vi "Striptest.vi"(1 "Simulation?":bool) -> ()   [LabVIEW 2013]
uses:
  InstrControl/SupplyControl/SupplyControl.lvclass
  InstrControl/Switching/Switching.lvclass
  InstrControl/ProbeStationControl/ProbeStationControl.lvclass
  InstrControl/LCRControl/LCRControl.lvclass
  general_VIs/globals/QC_MeasurementSetup.vi
  striptest/ProbePlan/ProbePlanParams.vi
  general_VIs/globals/QC_RunInformation.vi
  InstrControl/InstrumentSetup.vi
  <vilib>/regexp/Match Regular Expression.xnode
  InstrControl/InstrControl.lvclass
  InstrControl/ArduinoControl/ArduinoControl.lvclass
  <vilib>/Analysis/NI_AALBase.lvlib
panel:
  out "Tab Control":enum32{"Striptest Setup", "Striptest"}(tab)
  in  "Bias Voltage [V]":dbl=-150.0 format="%.1f"
  in  "Frequency [Hz] Setup":i32=1000 caption="Frequency [Hz]" format="%#.3p"
  in  "Minimum fraction\nof good strips":dbl=98.0 format="%.1g"
  in  "Quit":bool
  in  "Continue":bool
  in  "Measurement Configurations":bool
  in  "Pinholes Y/N":bool=TRUE
  in  "Capacitance Y/N":bool=TRUE
  in  "Resistance Y/N":bool=TRUE
  in  "Striptest SMU":string(combo)="Keithley 2410"
  in  "LCR Meter":string(combo)="WayneKerr 6440B"
  in  "Temperature":enum16{"Read Arduino", "Enter manually"}(ring)
  in  "Bias Supply":string(combo)="Keithley 2410"
  in  "Hardware Configurations":bool
  in  "DB Serial No. IN:":string caption="DB Serial No.:"
  in  "User:":string(combo)="Christoph"
  in  "Batch No. IN:":string caption="Batch No.:"
  in  "Device Category IN:":string(combo)="Short Strip" caption="Device Category:"
  in  "Sensor Serial No. IN:":string caption="Sensor Serial No.:"
  in  "From4":u16(ring)
  in  "From3":u16(ring)
  in  "From2":u16(ring)
  in  "From 1":u16(ring) caption="From"
  in  "To4":u16(ring)
  in  "To3":u16(ring)
  in  "To2":u16(ring)
  in  "To 1":u16(ring) caption="To"
  out "Region 1":string caption="Region"
  out "Region2":string
  out "Region3":string
  out "Region4":string
  in  "Enable1":bool
  in  "Enable4":bool
  in  "Enable2":bool
  in  "Enable3":bool
  in  "Pinhole Parameters IN":T1={"Base Voltage"=10.0, "Base Ramp [V/step]"=10.0, "Base Step [ms]"=1000, "High Voltage"=100.0, "High Ramp [V/step]"=100.0, "High Step [ms]"=1000} caption="Pinhole Measurement Parameters"
  in  "Manufacturer:":string(combo)="Hamamatsu"
  in  "Auto ReCheck":bool
  in  "Thresholds:":T2={"Current [nA]"=200.0, "Ccoupl Lo [pF/cm]"=20.0, "Ccoupl Hi [pF/cm]"=33.0, "Rbias Lo [MW]"=1.0, "Rbias Hi [MW]"=2.0}
  in  "Rolling\nCurrent Readout":bool=TRUE
  in  "settling\ndelay [ms]":i32=50
  in  "Pinhole Parameters":T1={"Base Voltage"=10.0, "Base Ramp [V/step]"=10.0, "Base Step [ms]"=1000, "High Voltage"=100.0, "High Ramp [V/step]"=100.0, "High Step [ms]"=1000}
  out "Bias On/Off:":bool
  in  "Auto quit &\nswitch off bias":bool
  out "Sensor No.:":string
  out "Device Category:":string
  out "DB Serial No.:":string
  out "Initiated:":string
  in  "ReCheck":bool
  in  "Save Data":bool
  in  "Abort":bool
  in  "Quit w/o saving":bool
  out "Probing Region:":string
  out "Probe Point:":string
  out "Current [nA]:":dbl
  out "Capacitance [pF]:":dbl
  out "Reistance [MW]:":dbl
  out "Last Probe at:":string
  out "Run Duration:":string
  out "Estimated Completion:":string
  out "Status:":string
  out "Probe Card Channels":i32=32
  in  "Show:":u16(ring)
  out "Defects":i32[][](graph)
  out "% OK:":dbl
  out "# total defects:":i32
  out "# probed":i32
  out "Bad Strip List":i32[](array[numeric])
  out "defect type array":i32[](array[numeric])
  out "Resistance [MW]":cluster{u32, i32, "Array OUT":dbl[]}(graph)
  out "Capacitance [pF]":cluster{u32, i32, "Array OUT":dbl[]}(graph)
  out "Current [nA]":cluster{u32, i32, "Array OUT":dbl[]}(graph)
  out "Current Reference 100V":dbl[](array[numeric])
  out "Current Reference 10V":dbl[](array[numeric])
  out "Single Needle":bool
  out "Z profile":i32[][](array[numeric])
  out "Start Temperature [°C]":dbl
  out "Last Temperature [°C]":dbl
  out "disabled channels":i32[](array[numeric])
  out "Module failed/passed":bool
  out "probe points per region":i32[](array[numeric])
  out "min scale array":i32[](array[numeric])
  out "max scale array":i32[](array[numeric])
  out "total strip number":u32
  out "Region Indices":i32[](array[numeric])
  out "Current Bias Voltage [V]":dbl
  out "Temperature Progression":T3
  # "University of \nCambridge"
  # "Sensor QC: Striptest"
  # "Current [nA]"
  # "Statistical information:"
  # "Pinholes:"
  # "Capacitance [pF]"
  # "Punchthroughs:"
  # "Shorts:"
  # "Opens:"
  # "Rpoly:"
  # "Resistance [MW]"
  # "Implant:"
  # "Current segment:"
  # "Ok  Pinhole at base  Pinhole after ramp  Short  Open  Rbias"
  # "Probe Range"
  # "Measurement Configuration"
  # "Hardware"
  # "DUT Description"
  # "Tests Included"
  # "Current status:"
  # "Measurement parameters:"
  # "DUT & Test Description:"
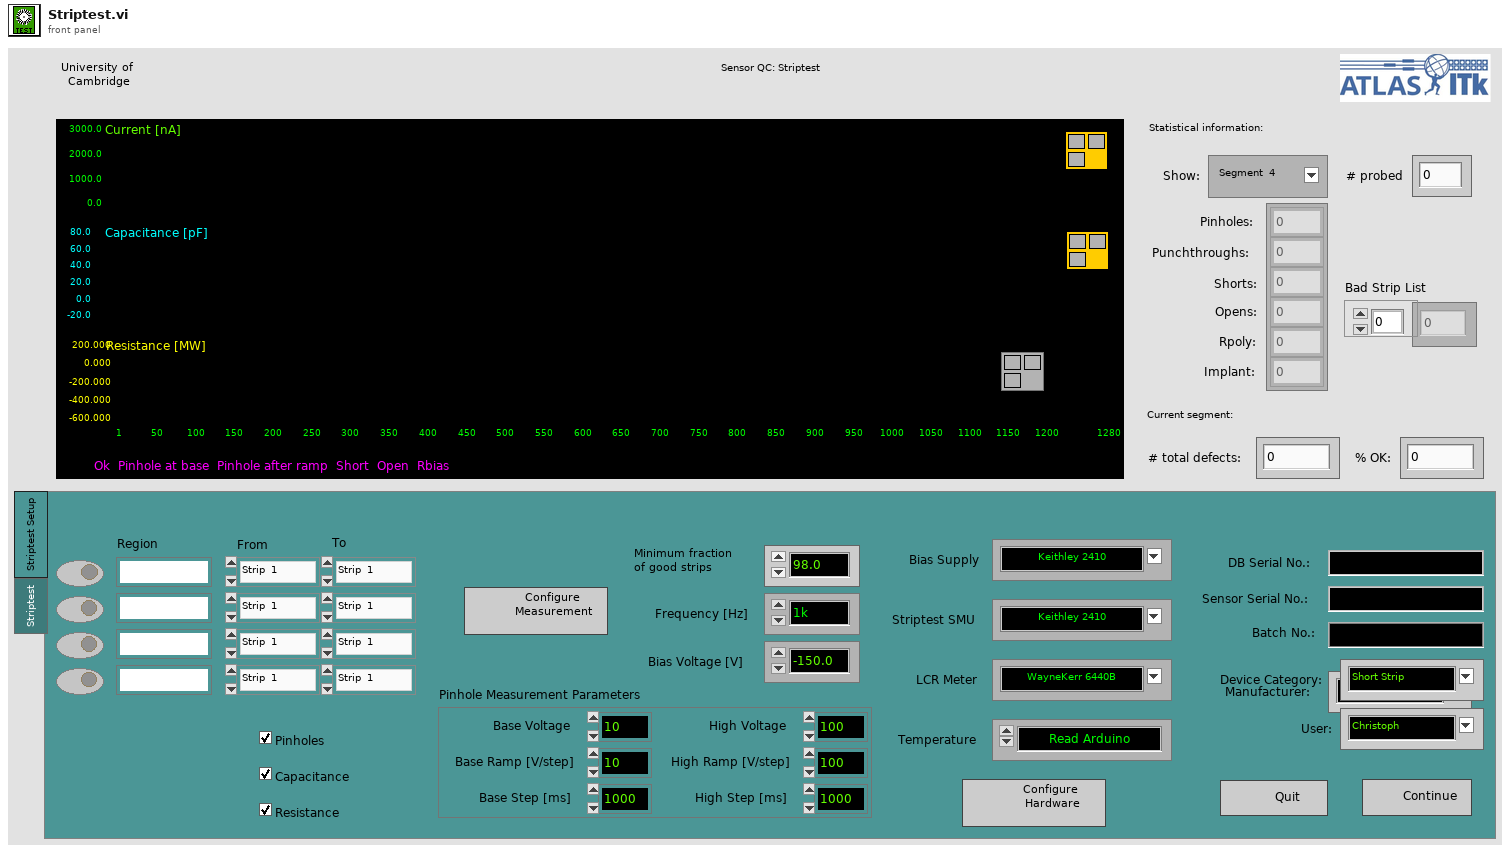
[diagram p1: front panel]
types:
  T1 = cluster{"Base Voltage":dbl, "Base Ramp [V/step]":dbl, "Base Step [ms]":i32, "High Voltage":dbl, "High Ramp [V/step]":dbl, "High Step [ms]":i32}
  T2 = cluster{"Current [nA]":dbl, "Ccoupl Lo [pF/cm]":dbl, "Ccoupl Hi [pF/cm]":dbl, "Rbias Lo [MW]":dbl, "Rbias Hi [MW]":dbl}
  T3 = cluster{"Time Array":string[], "Temperature Array [°C]":dbl[], "Humidity Array [RH %]":dbl[]}
  T4 = enum16{"Supply", "LCR", "Multimeter", "Switching"}
  T5 = enum16{"Reset", "Ground", "Striptest SMU", "Striptest LCR", "IV", "CV", "Interstrip Cap", "Interstrip Res"}
  T6 = enum16{"Reference measurement", "Baseline correcetion 10V", "Baseline correcetion 100V", "Nothing"}
  T7 = cluster{"Bias Supply":refnum<class "SupplyControl.lvclass">, "SMU":refnum<class "SupplyControl.lvclass">, "LCR":refnum<class "LCRControl.lvclass">, "Probe Card Channels":i32, "Bias Voltage [V]":dbl, "First strip":i32, "Last strip":i32, "Base Voltage [V]":dbl, "Base Ramp Step [V]":dbl, "Base Ramp Interval [ms]":u32, "High Voltage [V]":dbl, "High Ramp Step [V]":dbl, "High Ramp Interval [ms]":u32, "AC frequency [Hz]":i32, "AC amplitude [V]":dbl, "RC Configuration":u16, "Single Needle":bool, "Temperature Readout":enum16{"Read Arduino", "Enter manually"}, "Arduino":refnum<class "ArduinoControl.lvclass">, "Fraction of good strips [%]":dbl, "ProbeStation":refnum<class "ProbeStationControl.lvclass">, "Switching":refnum<class "Switching.lvclass">, "Matrix used?":bool, "Matrix X Channels":cluster{"Bias Supply / SMU LO":i32, "Bias Supply / SMU HI":i32, "CV Box LO":i32, "CV Box HI":i32, "CV Box LO IN":i32, "CV Box HI IN":i32, "Volt meter LO":i32, "Volt meter HI":i32, "Mux1 C1":i32, "Mux1 C2":i32, "Mux2 C1":i32, "Mux2 C2":i32}, "Pinholes Y/N":bool, "Capacitance Y/N":bool, "Resistance Y/N":bool, "Bias Supply Name":string, "SMU Name":string, "LCR Name":string}
  T8 = cluster{"Sensor Serial No.:":string, "Wafer Serial No.:":string, "Batch:":string, "Manufacturer:":string, "Device Category:":string, "Database Serial No.:":string, "Date Initiated:":string, "Time Initiated:":string, "Test":string, "Instruments used:":string, "Probeplan used:":string, "End of Run comment:":string, "User:":string}
  T9 = cluster{"Institute":string, "Manufacturers":string[], "Devices":string[], "Serialnumbers Lookup DB":string, "Data directory":string, "Backup & screenshot directory":string, "List of known users":string[], "Measurement switch not used":bool, "Measurement Switch":string, "DUT Switch":string}
  T10 = cluster{"Strip Number OUT":i32, "X0":i32, "Y0":i32, "X1":i32, "Y1":i32, "Xref":dbl, "Yref":dbl, "ProbePlan type":u32, "Inner pads offset":ext, "Outer pads offset":ext, "l_inner":ext, "l_outer":ext, "strip numbering":u16, "Device Orientation":ext, "Stagger offset":i32, "Yoffset":dbl, "Strip pitch":dbl, "Fiducail separation":dbl, "Radius":ext, "Relative strip angles":dbl, "Probeplan description":string, "ProbePlan array":cluster{"Region":string, "ProbePoints":cluster{"X":dbl, "Y":dbl, "Label":string, "CardViable?":bool}[]}[], "Test ProbePoints":cluster{"Regions Enabled":bool[], "From index":u32[], "To index":u32[]}}
  T11 = cluster{"Region":string, "ProbePoints":cluster{"X":dbl, "Y":dbl, "Label":string, "CardViable?":bool}[]}[]
  T12 = cluster{"VISA address":refnum<visa-resource-name>, "T sensor":enum16{"SHT", "DS"}, "Arduino":refnum<class "ArduinoControl.lvclass">}
  T13 = cluster{"X":dbl, "Y":dbl, "Label":string, "CardViable?":bool}[]
  T14 = cluster{"X":dbl, "Y":dbl, "Label":string, "CardViable?":bool}
  T15 = cluster{"pass Rate in %":dbl, "Bad channel list":i32[], "No of bad strips":i32, "Defect description list":i32[], "Number of defects per category":i32[], "Defect lists":string[], "No of channels":i32, "Defect Flag array OUT":i32[][]}
  T16 = cluster{"Hi Cap":dbl, "Lo Cap":dbl, "Current threshold":dbl, "Lo R":dbl, "Hi R":dbl}
  T17 = enum16{"Reset", "Read Array", "Read Element", "Write Element", "Write Array", "Add Element", "Add Array"}
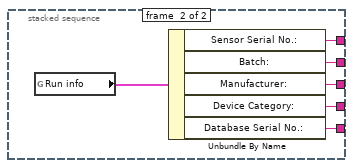
[diagram p2: hidden frame]
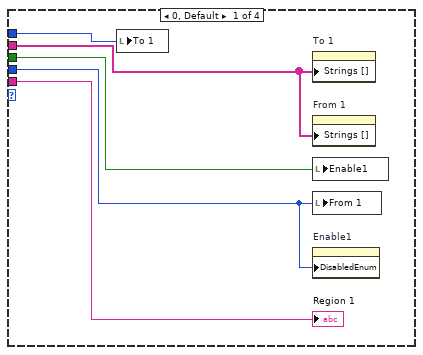
[diagram p3: hidden frame]
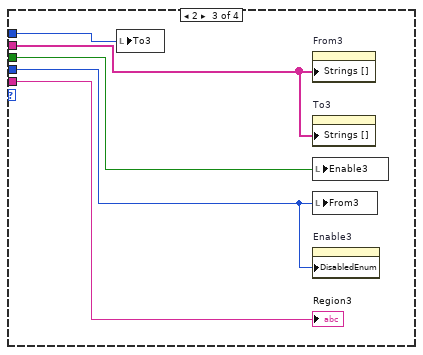
[diagram p4: hidden frame]
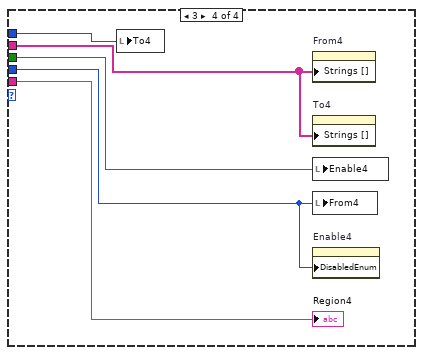
[diagram p5: hidden frame]
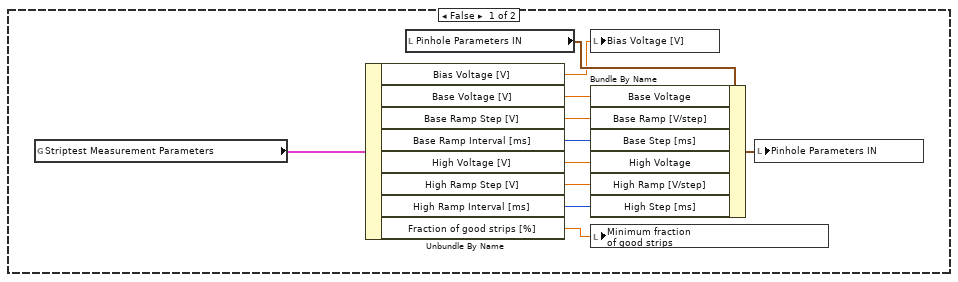
[diagram p7: hidden frame]
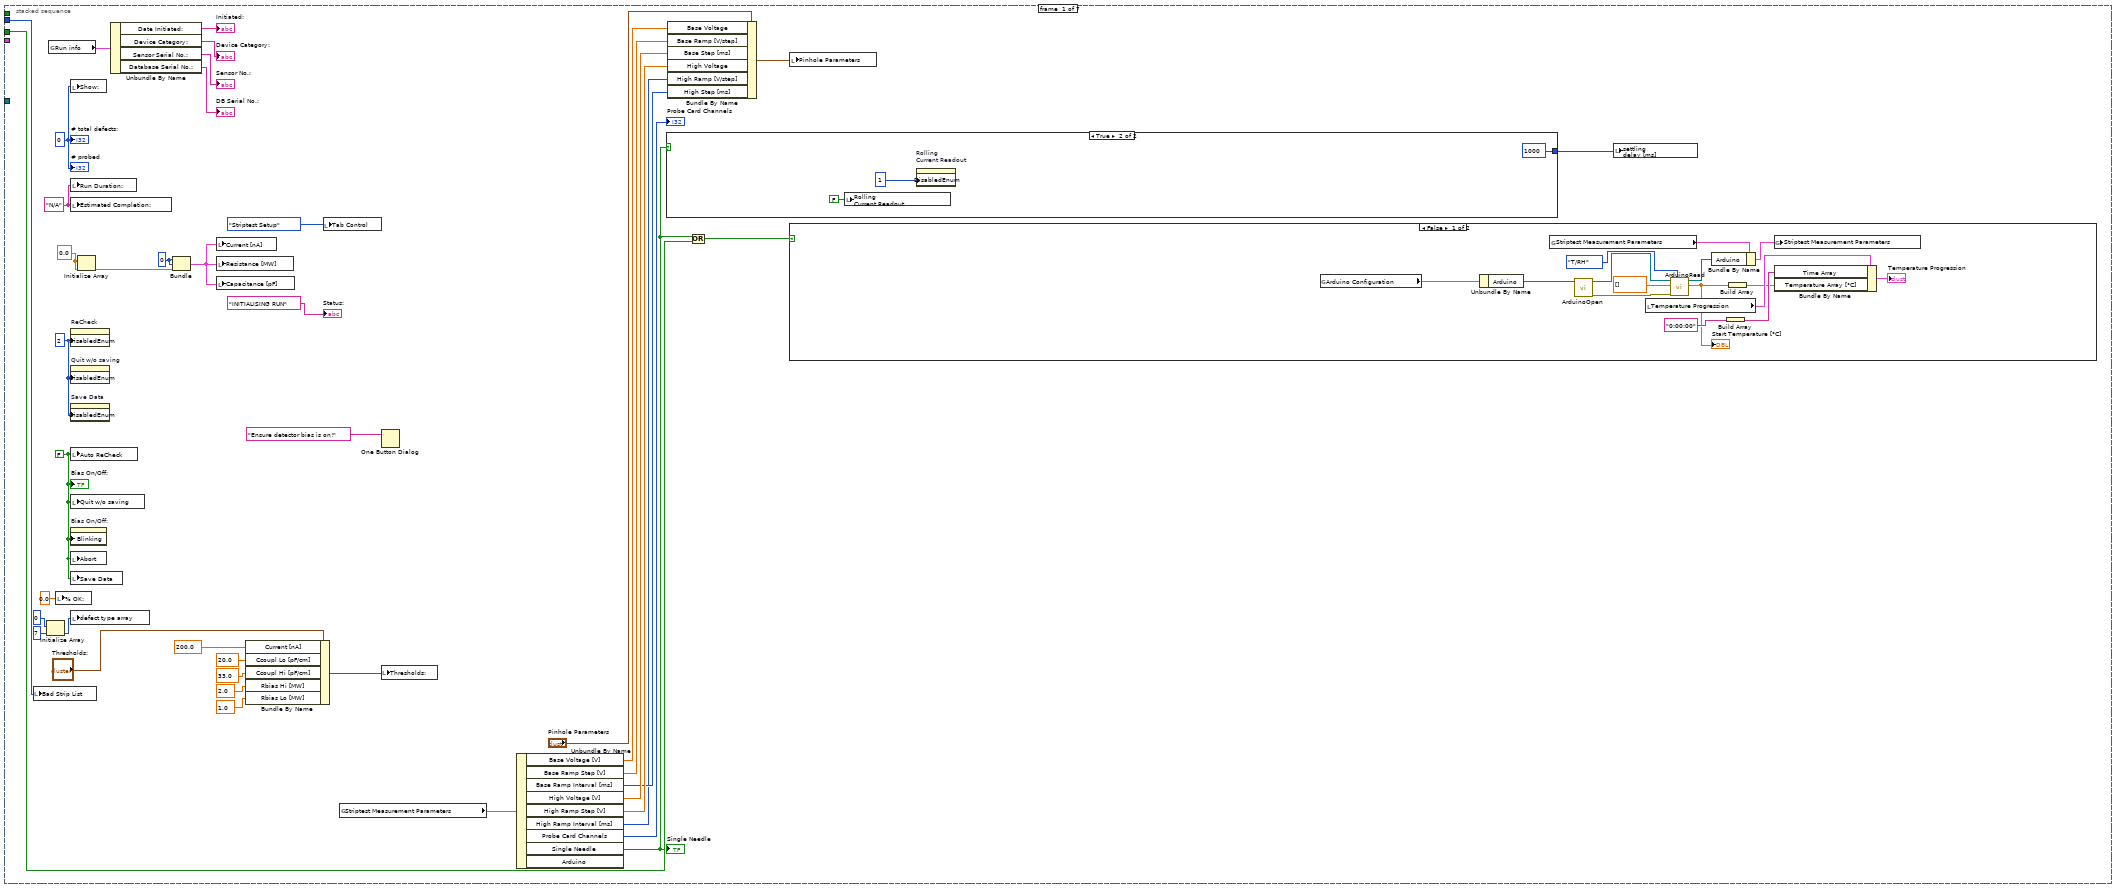
[diagram p10: hidden frame]
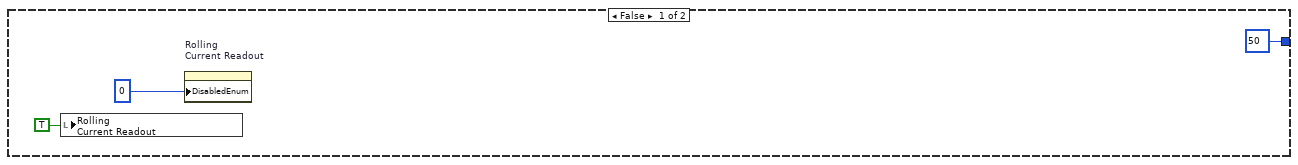
[diagram p11: hidden frame]
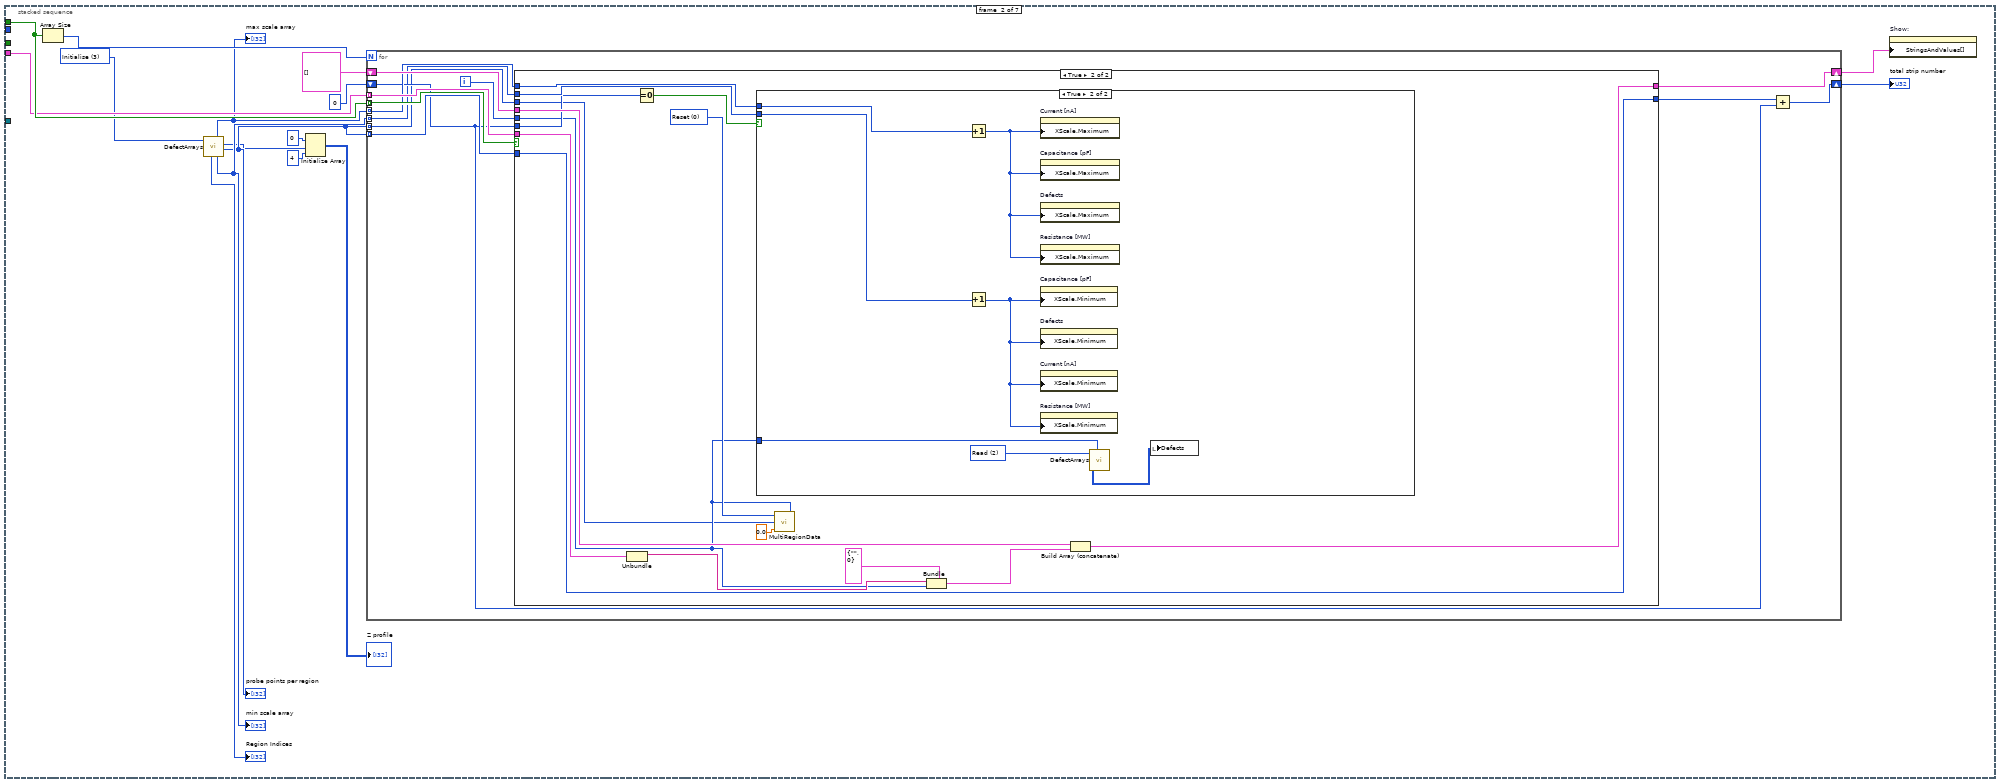
[diagram p13: hidden frame]
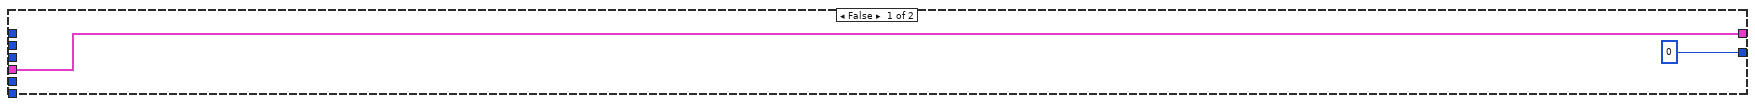
[diagram p14: hidden frame]
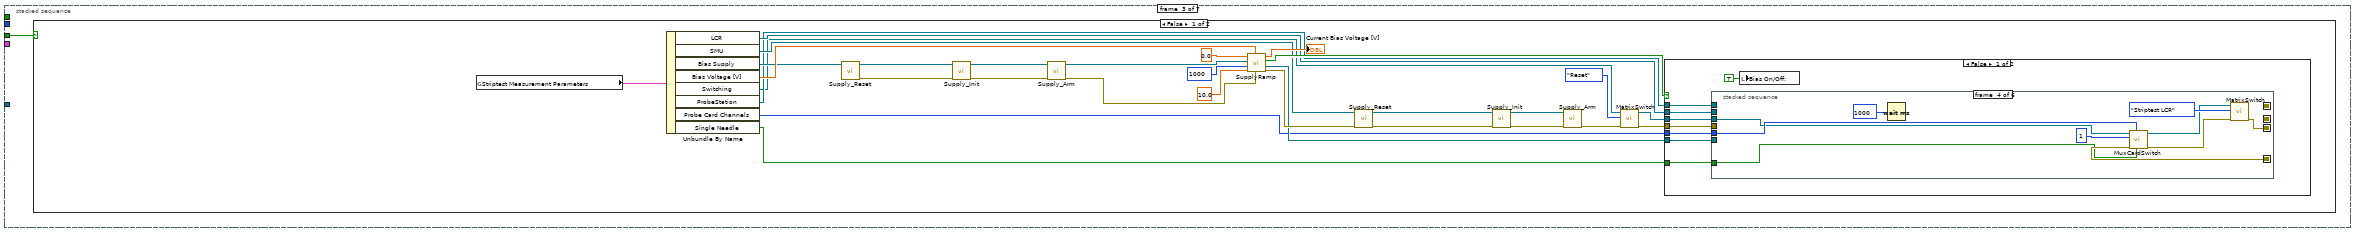
[diagram p16: hidden frame]
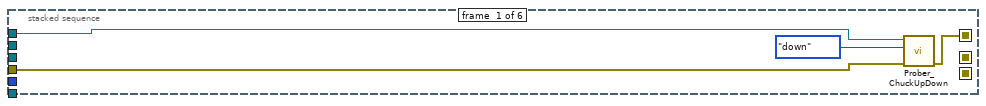
[diagram p17: hidden frame]
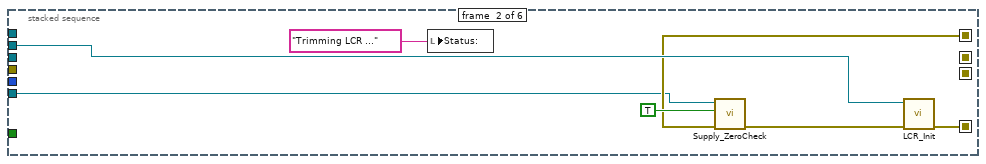
[diagram p18: hidden frame]
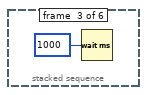
[diagram p19: hidden frame]
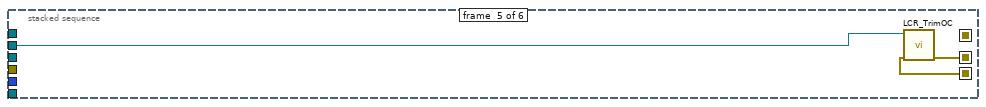
[diagram p20: hidden frame]
diagram:
  n1 = stacked-sequence {
    frame #0 {
      # "Striptest setup"
      n2 = flat-sequence {
        frame #0 {
          w1 = TRUE
          w3 = ""
          w4 = 2
          w5 = FALSE
          n3 = local write "Enable2"(w5) -> ()
          n4 = local write "Enable1"(w5) -> ()
          n5 = local write "Enable3"(w5) -> ()
          n6 = local write "Enable4"(w5) -> ()
          n7 = property on="Enable4" class="Bool (strict)"("DisabledEnum"=w4) -> ()  [unwired: 2 in, 2 out]
          n8 = property on="Enable1" class="Bool (strict)"("DisabledEnum"=w4) -> ()  [unwired: 2 in, 2 out]
          n9 = property on="Enable2" class="Bool (strict)"("DisabledEnum"=w4) -> ()  [unwired: 2 in, 2 out]
          n10 = property on="Enable3" class="Bool (strict)"("DisabledEnum"=w4) -> ()  [unwired: 2 in, 2 out]
          n11 = local write "Region 1"(w3) -> ()
          n12 = local write "Region2"(w3) -> ()
          n13 = local write "Region3"(w3) -> ()
          n14 = local write "Region4"(w3) -> ()
          n15 = call "SelectStriptestProber.vi"() -> ("error out"=w6:errorcluster, "ProbeStationControl out"=w7:refnum<class "ProbeStationControl.lvclass">)  [unwired: 10 in]
          n16 = global read "QC_MeasurementSetup.vi" "Striptest Measurement Parameters"() -> (w9:T7)
          n17 = call "InitialiseProbeplan.vi"("error in (no error)"=w6, "ProbeStationControl in"=w7) -> ()  [unwired: 8 in, 2 out]
          n18 = Bundle By Name(cluster=w9, "ProbeStation"=w7) -> (w8:T7)
          n19 = global write "QC_MeasurementSetup.vi" "Striptest Measurement Parameters"(w8) -> ()
          n20 = call "GetLocalConfiguration.vi"() -> ()  [unwired: 3 in, 1 out]
          n21 = call "GetGlobalDefaultConfiguration.vi"("DO NOT override instruments"=w1, "Read defaults?"=w1) -> ()  [unwired: 1 in, 1 out]
          "Tab Control" <- enum32{"Striptest Setup", "Striptest"}."Striptest Setup" ("Tab Control")
        }
        frame #1 {
          n22 = stacked-sequence {
            tunnel: [_ w54] -> w12
            tunnel: [_ w53] -> w13
            tunnel: [_ w52] -> w14
            tunnel: [_ w51] -> w15
            tunnel: [_ w49] -> w16
            frame #0 {
              n23 = call "SerialNo.vi"() -> ()  [unwired: 5 in, 1 out]
            }
            frame #1 {
              n24 = global read "QC_RunInformation.vi" "Run info"() -> (w50:T8)
              n25 = Unbundle By Name(w50) -> ("Sensor Serial No.:"=w54:string, "Batch:"=w53:string, "Manufacturer:"=w52:string, "Device Category:"=w51:string, "Database Serial No.:"=w49:string)
            }
          }
          n26 = global read "QC_RunInformation.vi" "Run info"() -> (w38:T8)
          n27 = Bundle By Name(cluster=w38, "Test"="Striptest") -> (w40:T8)
          n28 = call "InstrumentNames.vi"("Instrument type"=T4."Supply") -> ("error out"=w42:errorcluster, "Instrument names"=w44:string[])  [unwired: 9 in]
          n29 = property on="Bias Supply" class="CmbBox"("Strings[]"=w44) -> ()  [unwired: 2 in, 2 out]
          n30 = property on="Striptest SMU" class="CmbBox"("Strings[]"=w44) -> ()  [unwired: 2 in, 2 out]
          n31 = global write "QC_RunInformation.vi" "Run info"(w40) -> ()
          n32 = global read "QC_RunInformation.vi" "LocalConfiguration"() -> (w37:T9)
          n33 = global read "ProbePlanParams.vi" "ProbePlan Parameters IN"() -> (w48:T10)
          n34 = Unbundle By Name(w37) -> ("List of known users"=w35:string[], "Devices"=w11:string[], "Manufacturers"=w10:string[])
          n35 = call "InstrumentNames.vi"("error in (no error)"=w42, "Instrument type"=T4."LCR") -> ("Instrument names"=w41:string[])  [unwired: 8 in, 1 out]
          n36 = global read "QC_MeasurementSetup.vi" "Striptest Measurement Parameters"() -> (w34:T7)
          n37 = property on="LCR Meter" class="CmbBox"("Strings[]"=w41) -> ()  [unwired: 2 in, 2 out]
          n38 = property on="Device Category IN:" class="CmbBox"("Strings[]"=w11) -> ()  [unwired: 2 in, 2 out]
          n39 = property on="Manufacturer:" class="CmbBox"("Strings[]"=w10) -> ()  [unwired: 2 in, 2 out]
          n40 = local write "Sensor Serial No. IN:"(w12) -> ()
          n41 = local write "Batch No. IN:"(w13) -> ()
          n42 = local write "Manufacturer:"(w14) -> ()
          n43 = local write "Device Category IN:"(w15) -> ()
          n44 = local write "DB Serial No. IN:"(w16) -> ()
          n45 = Unbundle By Name(w48) -> ("ProbePlan array"=w47:T11)
          n46 = property on="User:" class="CmbBox"("Strings[]"=w35, "AllowUndefStrs"=TRUE) -> ()  [unwired: 2 in, 2 out]
          n47 = Array Size(array=w47) -> (size(s)=w46:i32)
          n48 = for {
            N: w46 -> [_]
            tunnel: w47 -> [w56]
            tunnel: w47 -> [w60] mode=indexing
            i -> [w63]
            n49 = Unbundle(w60) -> ("Region"=w59:string)  [unwired: 1 out]
            n50 = call "GetLabels.vi"("Array"=w56) -> ("Strip Labels"=w55:string[])  [unwired: 3 out]
            n51 = Array Size(array=w55) -> (size(s)=w58:i32)
            n52 = Decrement(x=w58) -> (x-1=w57:i32)
            n53 = case shown="1" w63 {
              tunnel: TRUE -> [w68 w72 w78 w83]
              tunnel: 0 -> [w64 w70 w74 w80]
              tunnel: w59 -> [w66 w71 w76 w81]
              tunnel: w55 -> [w65 w69 w75 w79]
              tunnel: w57 -> [w67 w73 w77 w82]
              frame 0, Default {
                n54 = local write "To 1"(w67) -> ()
                n55 = property on="To 1" class="Ring (strict)"("Strings []"=w65) -> ()  [unwired: 2 in, 2 out]
                n56 = property on="From 1" class="Ring (strict)"("Strings []"=w65) -> ()  [unwired: 2 in, 2 out]
                n57 = local write "Enable1"(w68) -> ()
                n58 = local write "From 1"(w64) -> ()
                n59 = property on="Enable1" class="Bool (strict)"("DisabledEnum"=w64) -> ()  [unwired: 2 in, 2 out]
                "Region 1" <- w66
              }
              frame 1 {
                n60 = local write "To2"(w73) -> ()
                n61 = property on="From2" class="Ring (strict)"("Strings []"=w69) -> ()  [unwired: 2 in, 2 out]
                n62 = property on="To2" class="Ring (strict)"("Strings []"=w69) -> ()  [unwired: 2 in, 2 out]
                n63 = local write "Enable2"(w72) -> ()
                n64 = local write "From2"(w70) -> ()
                n65 = property on="Enable2" class="Bool (strict)"("DisabledEnum"=w70) -> ()  [unwired: 2 in, 2 out]
                "Region2" <- w71
              }
              frame 2 {
                n66 = local write "To3"(w77) -> ()
                n67 = property on="From3" class="Ring (strict)"("Strings []"=w75) -> ()  [unwired: 2 in, 2 out]
                n68 = property on="To3" class="Ring (strict)"("Strings []"=w75) -> ()  [unwired: 2 in, 2 out]
                n69 = local write "Enable3"(w78) -> ()
                n70 = local write "From3"(w74) -> ()
                n71 = property on="Enable3" class="Bool (strict)"("DisabledEnum"=w74) -> ()  [unwired: 2 in, 2 out]
                "Region3" <- w76
              }
              frame 3 {
                n72 = local write "To4"(w82) -> ()
                n73 = property on="From4" class="Ring (strict)"("Strings []"=w79) -> ()  [unwired: 2 in, 2 out]
                n74 = property on="To4" class="Ring (strict)"("Strings []"=w79) -> ()  [unwired: 2 in, 2 out]
                n75 = local write "Enable4"(w83) -> ()
                n76 = local write "From4"(w80) -> ()
                n77 = property on="Enable4" class="Bool (strict)"("DisabledEnum"=w80) -> ()  [unwired: 2 in, 2 out]
                "Region4" <- w81
              }
            }
          }
          n78 = Unbundle By Name(w34) -> ("Probe Card Channels"=w33:i32, "Bias Voltage [V]"=w24:dbl, "Base Voltage [V]"=w30:dbl, "Base Ramp Step [V]"=w29:dbl, "Base Ramp Interval [ms]"=w28:u32, "High Voltage [V]"=w27:dbl, "High Ramp Step [V]"=w26:dbl, "High Ramp Interval [ms]"=w25:u32, "Single Needle"=w23:bool, "Temperature Readout"=w22:enum16{"Read Arduino", "Enter manually"}, "Fraction of good strips [%]"=w21:dbl, "AC frequency [Hz]"=w20:i32, "Pinholes Y/N"=w19:bool, "Capacitance Y/N"=w18:bool, "Resistance Y/N"=w17:bool)
          n79 = local read "Pinhole Parameters IN"() -> (w32:T1)
          n80 = Bundle By Name(cluster=w32, "Base Voltage"=w30, "Base Ramp [V/step]"=w29, "Base Step [ms]"=w28, "High Voltage"=w27, "High Ramp [V/step]"=w26, "High Step [ms]"=w25) -> (w31:T1)
          n81 = local write "Probe Card Channels"(w33) -> ()
          n82 = local write "Bias Voltage [V]"(w24) -> ()
          n83 = local write "Single Needle"(w23) -> ()
          n84 = local write "Temperature"(w22) -> ()
          n85 = local write "Minimum fraction\nof good strips"(w21) -> ()
          n86 = local write "Frequency [Hz] Setup"(w20) -> ()
          n87 = local write "Pinholes Y/N"(w19) -> ()
          n88 = local write "Capacitance Y/N"(w18) -> ()
          n89 = local write "Resistance Y/N"(w17) -> ()
          n90 = local write "Pinhole Parameters IN"(w31) -> ()
        }
        frame #2 {
          n91 = while {
            shift-right: [w87] -> _
            shift-left: FALSE -> [w89]
            stop <- "Continue" stop-if-true
            n92 = Stop(stop? (T)="Quit") -> ()
            n93 = local read "Sensor Serial No. IN:"() -> (w95:string)
            n94 = local read "DB Serial No. IN:"() -> (w93:string)
            n95 = local read "Batch No. IN:"() -> (w94:string)
            n96 = Empty String/Path?(string/path=w95) -> (empty?=w92:bool)
            n97 = Empty String/Path?(string/path=w94) -> (empty?=w91:bool)
            n98 = Empty String/Path?(string/path=w93) -> (empty?=w90:bool)
            n99 = case shown="True" "Measurement Configurations" {
              frame False {
              }
              frame True {
                n100 = Two Button Dialog(message="With this, you will change QC measurement parameters defined by the collaboration!\n\nDo you really wish to continue?", 2:"YES") -> (T button?=w101:bool)  [unwired: 1 in]
                n101 = case shown="True" w101 {
                  frame False {
                    n102 = global read "QC_MeasurementSetup.vi" "Striptest Measurement Parameters"() -> (w114:T7)
                    n103 = Unbundle By Name(w114) -> ("Bias Voltage [V]"=w104:dbl, "Base Voltage [V]"=w111:dbl, "Base Ramp Step [V]"=w110:dbl, "Base Ramp Interval [ms]"=w109:u32, "High Voltage [V]"=w108:dbl, "High Ramp Step [V]"=w107:dbl, "High Ramp Interval [ms]"=w106:u32, "Fraction of good strips [%]"=w105:dbl)
                    n104 = local read "Pinhole Parameters IN"() -> (w113:T1)
                    n105 = local write "Bias Voltage [V]"(w104) -> ()
                    n106 = Bundle By Name(cluster=w113, "Base Voltage"=w111, "Base Ramp [V/step]"=w110, "Base Step [ms]"=w109, "High Voltage"=w108, "High Ramp [V/step]"=w107, "High Step [ms]"=w106) -> (w112:T1)
                    n107 = local write "Minimum fraction\nof good strips"(w105) -> ()
                    n108 = local write "Pinhole Parameters IN"(w112) -> ()
                  }
                  frame True {
                    n109 = global read "QC_MeasurementSetup.vi" "Striptest Measurement Parameters"() -> (w125:T7)
                    n110 = Unbundle By Name("Pinhole Parameters IN") -> ("Base Voltage"=w121:dbl, "Base Ramp [V/step]"=w120:dbl, "Base Step [ms]"=w119:i32, "High Voltage"=w118:dbl, "High Ramp [V/step]"=w117:dbl, "High Step [ms]"=w116:i32)
                    n111 = Bundle By Name(cluster=w125, "Bias Voltage [V]"="Bias Voltage [V]", "Base Voltage [V]"=w121, "Base Ramp Step [V]"=w120, "Base Ramp Interval [ms]"=w119, "High Voltage [V]"=w118, "High Ramp Step [V]"=w117, "High Ramp Interval [ms]"=w116, "Fraction of good strips [%]"="Minimum fraction\nof good strips") -> (w124:T7)
                    n112 = global write "QC_MeasurementSetup.vi" "Striptest Measurement Parameters"(w124) -> ()
                  }
                }
              }
            }
            n113 = case shown="True" "Hardware Configurations" {
              tunnel: [w126 w127] -> w87
              tunnel: w89 -> [w126 _]
              frame False {
              }
              frame True {
                n114 = call "HardwareConfiguration.vi"() -> ("configured?"=w127:bool)  [unwired: 11 in]
              }
            }
            n115 = Compound Arithmetic op=OR(w92, w91, w90) -> (invert w96:bool)
            n116 = Select(t=0, s=w96, f=2) -> (s? t:f=w86:i32)
            n117 = property on="Continue" class="Bool"("DisabledEnum"=w86) -> ()  [unwired: 2 in, 2 out]
          }
        }
        frame #3 {
          w148 = TRUE
          w155 = T4."Supply" ("Instrument type")
          n118 = call "InstrumentSelection.vi"("Verify GPIB address"=w148, "Instrument type"=w155, "Instrument name IN"="Bias Supply") -> ("error out"=w161:errorcluster, "Instrument name OUT"=w135:string, "Supply"=w156:refnum<class "SupplyControl.lvclass">)  [unwired: 3 in, 3 out]
          n119 = call "InstrumentSelection.vi"("error in (no error)"=w161, "Verify GPIB address"=w148, "Instrument type"=w155, "Instrument name IN"="Striptest SMU") -> ("error out"=w149:errorcluster, "Instrument name OUT"=w134:string, "Supply"=w153:refnum<class "SupplyControl.lvclass">)  [unwired: 2 in, 3 out]
          n120 = global read "ProbePlanParams.vi" "ProbePlan Parameters IN"() -> (w184:T10)
          n121 = Build Array("Enable1", "Enable2", "Enable3", "Enable4") -> (w182:bool[])
          n122 = Build Array("From 1", "From2", "From3", "From4") -> (w181:u16[])
          n123 = Build Array("To 1", "To2", "To3", "To4") -> (w180:u16[])
          n124 = call "InstrumentSelection.vi"("error in (no error)"=w149, "Verify GPIB address"=w148, "Instrument type"=T4."LCR", "Instrument name IN"="LCR Meter") -> ("error out"=w150:errorcluster, "Instrument name OUT"=w133:string, "LCR"=w152:refnum<class "LCRControl.lvclass">)  [unwired: 2 in, 3 out]
          n125 = global read "QC_MeasurementSetup.vi" "Striptest Measurement Parameters"() -> (w158:T7)
          n126 = Bundle By Name(cluster=w184, "Test ProbePoints.Regions Enabled"=w182, "Test ProbePoints.From index"=w181, "Test ProbePoints.To index"=w180) -> (w183:T10)
          n127 = Unbundle By Name(w184) -> ("Probeplan description"=w139:string)
          n128 = Format Into String(format string="%s, %s, %s", w135, w134, w133) -> (resulting string=w132:string)  [unwired: 2 in, 1 out]
          n129 = call "InstrumentSelection.vi"("error in (no error)"=w150, "Verify GPIB address"=w148, "Instrument type"=T4."Switching", "Instrument name IN"="Pickering Matrix") -> ("Switching"=w151:refnum<class "Switching.lvclass">)  [unwired: 2 in, 5 out]
          n130 = global read "QC_RunInformation.vi" "Run info"() -> (w159:T8)
          n131 = Get Date/Time String(date format (0)=enum16{"short", "long", "abbreviated"}."abbreviated", want seconds? (F)=TRUE) -> (date string=w141:string, time string=w140:string)  [unwired: 1 in]
          n132 = Bundle By Name(cluster=w158, "Bias Supply"=w156, "SMU"=w153, "LCR"=w152, "Switching"=w151, "Temperature Readout"="Temperature", "AC frequency [Hz]"="Frequency [Hz] Setup", "Pinholes Y/N"="Pinholes Y/N", "Capacitance Y/N"="Capacitance Y/N", "Resistance Y/N"="Resistance Y/N") -> (w157:T7)
          n133 = global write "ProbePlanParams.vi" "ProbePlan Parameters IN"(w183) -> ()
          n134 = global write "QC_MeasurementSetup.vi" "Striptest Measurement Parameters"(w157) -> ()
          n135 = Bundle By Name(cluster=w159, "Sensor Serial No.:"="Sensor Serial No. IN:", "Batch:"="Batch No. IN:", "Manufacturer:"="Manufacturer:", "Device Category:"="Device Category IN:", "Database Serial No.:"="DB Serial No. IN:", "Date Initiated:"=w141, "Time Initiated:"=w140, "Instruments used:"=w132, "Probeplan used:"=w139, "User:"="User:") -> (w167:T8)
          n136 = global write "QC_RunInformation.vi" "Run info"(w167) -> ()
        }
      }
    }
    frame #1 {
      # "Striptest measurement procedure"
      n137 = global read "QC_MeasurementSetup.vi" "Striptest Measurement Parameters"() -> (w185:T7)
      n138 = global read "ProbePlanParams.vi" "ProbePlan Parameters IN"() -> (w192:T10)
      n139 = Unbundle By Name(w192) -> ("Test ProbePoints.Regions Enabled"=w188:bool[], "ProbePlan array"=w187:T11)
      n140 = Unbundle By Name(w185) -> ("ProbeStation"=w186:refnum<class "ProbeStationControl.lvclass">)
      n141 = Initialize Array(0) -> (w190:i32[])  [unwired: 1 in]
      n142 = stacked-sequence {
        tunnel: w190 -> [w213 _ _ _ w415 _ _]
        tunnel: "Simulation?" -> [w208 _ w308 w393 _ w1029 w1086]
        tunnel: w188 -> [_ w270 _ _ w418 _ w1085]
        tunnel: w187 -> [_ w269 _ _ w416 _ _]
        tunnel: w186 -> [_ _ _ w391 _ w1028 _]
        frame #0 {
          w215 = "N/A"
          w210 = FALSE
          w223 = 2
          w216 = 0
          w233 = 0
          w232 = 0.0
          n143 = local write "Bad Strip List"(w213) -> ()
          n144 = Initialize Array(0, 7 ("Dimension Size")) -> (w211:i32[])
          n145 = global read "QC_RunInformation.vi" "Run info"() -> (w230:T8)
          n146 = local write "% OK:"(0.0) -> ()
          n147 = local write "Show:"(w216) -> ()
          n148 = local write "Run Duration:"(w215) -> ()
          n149 = local write "Estimated Completion:"(w215) -> ()
          n150 = property on="ReCheck" class="Bool"("DisabledEnum"=w223) -> ()  [unwired: 2 in, 2 out]
          n151 = property on="Quit w/o saving" class="Bool (strict)"("DisabledEnum"=w223) -> ()  [unwired: 2 in, 2 out]
          n152 = property on="Save Data" class="Bool (strict)"("DisabledEnum"=w223) -> ()  [unwired: 2 in, 2 out]
          n153 = local write "Auto ReCheck"(w210) -> ()
          n154 = local write "Quit w/o saving"(w210) -> ()
          n155 = property on="Bias On/Off:" class="Bool (strict)"("Blinking"=w210) -> ()  [unwired: 2 in, 2 out]
          n156 = local write "Abort"(w210) -> ()
          n157 = local write "Save Data"(w210) -> ()
          n158 = local write "defect type array"(w211) -> ()
          n159 = Initialize Array(w232, w232) -> (w234:dbl[])
          n160 = Unbundle By Name(w230) -> ("Date Initiated:"=→"Initiated:":string, "Device Category:"=→"Device Category:":string, "Sensor Serial No.:"=→"Sensor No.:":string, "Database Serial No.:"=→"DB Serial No.:":string)
          n161 = Bundle(w233, w233, w234) -> (w231:cluster{i32, i32, dbl[]})  [unwired: 1 in]
          n162 = local write "Current [nA]"(w231) -> ()
          n163 = local write "Resistance [MW]"(w231) -> ()
          n164 = local write "Capacitance [pF]"(w231) -> ()
          n165 = Bundle By Name(cluster="Thresholds:", "Current [nA]"=200.0 ("CapLo"), "Ccoupl Lo [pF/cm]"=20.0 ("CapLo"), "Ccoupl Hi [pF/cm]"=33.0 ("CapHi"), "Rbias Hi [MW]"=2.0 ("Rpolyhi"), "Rbias Lo [MW]"=1.0 ("RpolyLo")) -> (w221:T2)
          n166 = local write "Tab Control"(enum32{"Striptest Setup", "Striptest"}."Striptest Setup" ("Tab Control")) -> ()
          n167 = global read "QC_MeasurementSetup.vi" "Striptest Measurement Parameters"() -> (w196:T7)
          n168 = One Button Dialog(message="Ensure detector bias is on!") -> ()  [unwired: 1 in, 1 out]
          n169 = local write "Thresholds:"(w221) -> ()
          n170 = Unbundle By Name(w196) -> ("Base Voltage [V]"=w204:dbl, "Base Ramp Step [V]"=w205:dbl, "Base Ramp Interval [ms]"=w201:u32, "High Voltage [V]"=w202:dbl, "High Ramp Step [V]"=w203:dbl, "High Ramp Interval [ms]"=w200:u32, "Probe Card Channels"=→"Probe Card Channels":i32, "Single Needle"=w195:bool)  [unwired: 1 out]
          "Single Needle" <- w195
          n171 = case shown="True" w195 {
            tunnel: [50 1000] -> w197
            frame False {
              n172 = local write "Rolling\nCurrent Readout"(TRUE) -> ()
              n173 = property on="Rolling\nCurrent Readout" class="Bool (strict)"("DisabledEnum"=0) -> ()  [unwired: 2 in, 2 out]
            }
            frame True {
              n174 = local write "Rolling\nCurrent Readout"(FALSE) -> ()
              n175 = property on="Rolling\nCurrent Readout" class="Bool (strict)"("DisabledEnum"=1) -> ()  [unwired: 2 in, 2 out]
            }
          }
          n176 = Bundle By Name(cluster="Pinhole Parameters", "Base Voltage"=w204, "Base Ramp [V/step]"=w205, "Base Step [ms]"=w202, "High Voltage"=w203, "High Ramp [V/step]"=w200, "High Step [ms]"=w201) -> (w206:T1)
          n177 = Or(x=w195, y=w208) -> (x .or. y?=w207:bool)
          n178 = local write "Pinhole Parameters"(w206) -> ()
          n179 = case shown="False" w207 {
            frame False {
              n180 = global read "InstrumentSetup.vi" "Arduino Configuration"() -> (w255:T12)
              n181 = Unbundle By Name(w255) -> ("Arduino"=w247:refnum<class "ArduinoControl.lvclass">)
              n182 = global read "QC_MeasurementSetup.vi" "Striptest Measurement Parameters"() -> (w243:T7)
              n183 = call "ArduinoOpen.vi"("ArduinoControl in"=w247) -> ("error out"=w245:errorcluster, "ArduinoControl out"=w246:refnum<class "ArduinoControl.lvclass">)  [unwired: 9 in]
              n184 = local read "Temperature Progression"() -> (w254:T3)
              n185 = call "ArduinoRead.vi"("Arduino function"=enum16{"T/RH", "Interlock", "Edgesense"}."T/RH", "error in (no error)"=w245, "Temperature IN"=dbl[] [], "ArduinoControl in"=w246) -> ("Temperature [°C]"=w249:dbl, "ArduinoControl out"=w241:refnum<class "ArduinoControl.lvclass">)  [unwired: 2 in, 4 out]
              "Start Temperature [°C]" <- w249
              n186 = Bundle By Name(cluster=w243, "Arduino"=w241) -> (w242:T7)
              n187 = Build Array("0:00:00") -> (w250:string[])
              n188 = Build Array(w249) -> (w248:dbl[])
              n189 = global write "QC_MeasurementSetup.vi" "Striptest Measurement Parameters"(w242) -> ()
              n190 = Bundle By Name(cluster=w254, "Time Array"=w250, "Temperature Array [°C]"=w248) -> (→"Temperature Progression":T3)
            }
            frame True {
            }
          }
          n191 = local write "settling\ndelay [ms]"(w197) -> ()
          "# total defects:" <- w216
          "# probed" <- w216
          "Status:" <- "INITIALISING RUN"
          "Bias On/Off:" <- w210
        }
        frame #1 {
          w265 = u16 3 items=["Nothing", "Write", "Read", "Initialise"] ("action")
          n192 = Array Size(array=w270) -> (size(s)=w271:i32)
          n193 = call "DefectArrays.vi"("action"=w265) -> ("Region Indices"=→"Region Indices":i32[], "To"=w264:i32[], "max. No. of points in region"=w256:i32, "From"=w263:i32[], "No. of points in region"=w258:i32[])  [unwired: 2 in, 3 out]
          "max scale array" <- w264
          "min scale array" <- w263
          "probe points per region" <- w258
          n194 = Initialize Array(0, w256, 4) -> (→"Z profile":i32[][])
          n195 = for {
            N: w271 -> [_]
            tunnel: w270 -> [w283] mode=indexing
            shift-right: [w282] -> w268
            shift-left: cluster{string, i32}[] [] -> [w281]
            tunnel: w269 -> [w280] mode=indexing
            tunnel: w258 -> [w275] mode=indexing
            tunnel: w264 -> [w276] mode=indexing
            tunnel: w263 -> [w273] mode=indexing
            shift-right: [w277] -> w267
            shift-left: 0 -> [w274]
            tunnel: w258 -> [w272] mode=indexing
            i -> [w278]
            n196 = case shown="True" w283 {
              tunnel: w281 -> [w284 w299]
              tunnel: [w284 w298] -> w282
              tunnel: w280 -> [_ w300]
              tunnel: [0 w294] -> w279
              tunnel: w278 -> [_ w289]
              tunnel: w276 -> [_ w296]
              tunnel: w273 -> [_ w295]
              tunnel: w275 -> [_ w294]
              tunnel: w274 -> [_ w293]
              tunnel: w272 -> [_ w287]
              frame False {
              }
              frame True {
                w291 = u32 0 items=["Reset", "Read Array", "Read Element", "Write Element", "Write Array"] ("Action")
                n197 = Unbundle(w300) -> ("Region"=w290:string)  [unwired: 1 out]
                n198 = Equal To 0?(x=w293) -> (x = 0?=w297:bool)
                n199 = case shown="True" w297 {
                  tunnel: w296 -> [_ w302]
                  tunnel: w295 -> [_ w304]
                  tunnel: w289 -> [_ w305]
                  frame False {
                  }
                  frame True {
                    w307 = u16 2 items=["Nothing", "Write", "Read", "Initialise"] ("action")
                    n200 = Increment(x=w302) -> (x+1=w301:i32)
                    n201 = Increment(x=w304) -> (x+1=w303:i32)
                    n202 = property on="Current [nA]" class="WFGraph (strict)"("XScale.Maximum"=w301) -> ()  [unwired: 2 in, 2 out]
                    n203 = property on="Capacitance [pF]" class="WFGraph (strict)"("XScale.Maximum"=w301) -> ()  [unwired: 2 in, 2 out]
                    n204 = property on="Defects" class="IntGraph (strict)"("XScale.Maximum"=w301) -> ()  [unwired: 2 in, 2 out]
                    n205 = property on="Resistance [MW]" class="WFGraph (strict)"("XScale.Maximum"=w301) -> ()  [unwired: 2 in, 2 out]
                    n206 = property on="Capacitance [pF]" class="WFGraph (strict)"("XScale.Minimum"=w303) -> ()  [unwired: 2 in, 2 out]
                    n207 = property on="Defects" class="IntGraph (strict)"("XScale.Minimum"=w303) -> ()  [unwired: 2 in, 2 out]
                    n208 = property on="Current [nA]" class="WFGraph (strict)"("XScale.Minimum"=w303) -> ()  [unwired: 2 in, 2 out]
                    n209 = property on="Resistance [MW]" class="WFGraph (strict)"("XScale.Minimum"=w303) -> ()  [unwired: 2 in, 2 out]
                    n210 = call "DefectArrays.vi"("action"=w307, "Region Index"=w305) -> ("Defect array OUT"=w306:i32[][])  [unwired: 1 in, 7 out]
                    n211 = local write "Defects"(w306) -> ()
                  }
                }
                n212 = call "MultiRegionData.vi"("Action"=w291, "Array Size / Index"=w287, "Data IN"=0.0, "Region index"=w289) -> ()  [unwired: 2 in, 2 out]
                n213 = Bundle(cluster=cluster{string, i32} {"", 0}, w290, w289) -> (w288:cluster{string, i32})
                n214 = Build Array (concatenate)(w299, w288) -> (w298:cluster{string, i32}[])
              }
            }
            n215 = Add(x=w279, y=w274) -> (x+y=w277:i32)
          }
          "total strip number" <- w267
          n216 = property on="Show:" class="Ring (strict)"("StringsAndValues[]"=w268) -> ()  [unwired: 2 in, 2 out]
        }
        frame #2 {
          n217 = case shown="False" w308 {
            frame False {
              n218 = global read "QC_MeasurementSetup.vi" "Striptest Measurement Parameters"() -> (w337:T7)
              n219 = Unbundle By Name(w337) -> ("LCR"=w314:refnum<class "LCRControl.lvclass">, "SMU"=w315:refnum<class "SupplyControl.lvclass">, "Bias Supply"=w316:refnum<class "SupplyControl.lvclass">, "Bias Voltage [V]"=w326:dbl, "Switching"=w311:refnum<class "Switching.lvclass">, "ProbeStation"=w313:refnum<class "ProbeStationControl.lvclass">, "Probe Card Channels"=w310:i32, "Single Needle"=w309:bool)
              n220 = call-dynamic "Supply_Reset.vi"("SupplyControl in"=w316) -> ("error out"=w330:errorcluster, "SupplyControl out"=w333:refnum<class "SupplyControl.lvclass">)  [unwired: 9 in]
              n221 = call-dynamic "Supply_Init.vi"("error in (no error)"=w330, "SupplyControl in"=w333) -> ("error out"=w331:errorcluster, "SupplyControl out"=w332:refnum<class "SupplyControl.lvclass">)  [unwired: 8 in]
              n222 = call-dynamic "Supply_Arm.vi"("error in (no error)"=w331, "SupplyControl in"=w332) -> ("error out"=w328:errorcluster, "SupplyControl out"=w329:refnum<class "SupplyControl.lvclass">)  [unwired: 8 in]
              n223 = call "SupplyRamp.vi"("error in"=w328, "Requested Voltage"=w326, "Step Size"=10.0, "Step Delay"=1000, "Supply IN"=w329, "Starting Voltage"=0.0) -> ("error out"=w327:errorcluster, "Supply OUT"=w312:refnum<class "SupplyControl.lvclass">, "Compliance exceeded"=w320:bool, "Current Voltage"=→"Current Bias Voltage [V]":dbl)  [unwired: 2 in]
              n224 = call-dynamic "Supply_Reset.vi"("error in (no error)"=w327, "SupplyControl in"=w315) -> ("error out"=w324:errorcluster, "SupplyControl out"=w323:refnum<class "SupplyControl.lvclass">)  [unwired: 8 in]
              n225 = call-dynamic "Supply_Init.vi"("error in (no error)"=w324, "SupplyControl in"=w323) -> ("error out"=w325:errorcluster, "SupplyControl out"=w322:refnum<class "SupplyControl.lvclass">)  [unwired: 8 in]
              n226 = call-dynamic "Supply_Arm.vi"("error in (no error)"=w325, "SupplyControl in"=w322) -> ("error out"=w338:errorcluster)  [unwired: 8 in, 1 out]
              n227 = call-dynamic "MatrixSwitch.vi"("error in (no error)"=w338, "Action"=T5."Reset", "Switching in"=w311) -> ("error out"=w317:errorcluster, "Switching out"=w318:refnum<class "Switching.lvclass">)  [unwired: 6 in, 1 out]
              n228 = case shown="False" w320 {
                selector: w320 -> [_ w390]
                tunnel: w318 -> [w345 _]
                tunnel: w317 -> [w344 _]
                tunnel: w314 -> [w343 _]
                tunnel: w313 -> [w342 _]
                tunnel: w312 -> [w341 _]
                tunnel: w310 -> [w340 _]
                tunnel: w309 -> [w339 _]
                frame False {
                  n229 = stacked-sequence {
                    seq-local: [w348 _ _ _ _ _] -> [_ w353 _ _ _ _]
                    seq-local: [_ w357 _ _ _ _] -> [_ _ _ w363 _ _]
                    seq-local: [_ _ _ w364 _ _] -> [_ _ _ _ w371 _]
                    seq-local: [_ _ _ _ w369 _] -> [_ _ _ _ _ w376]
                    tunnel: w345 -> [_ _ _ w360 _ w377]
                    tunnel: w344 -> [w349 _ _ _ _ _]
                    tunnel: w343 -> [_ w356 _ _ w370 _]
                    tunnel: w342 -> [w347 _ _ _ _ _]
                    tunnel: w341 -> [_ w351 _ _ _ w378]
                    tunnel: w340 -> [_ _ _ w361 _ w373]
                    tunnel: w339 -> [_ _ _ w362 _ w372]
                    frame #0 {
                      n230 = call-dynamic "Prober_ChuckUpDown.vi"("error in (no error)"=w349, "Direction"=enum16{"up", "down"}."down", "ProbeStationControl in"=w347) -> ("error out"=w348:errorcluster)  [unwired: 6 in, 2 out]
                    }
                    frame #1 {
                      n231 = local write "Status:"("Trimming LCR ..." ("STATUS 1")) -> ()
                      n232 = call-dynamic "Supply_ZeroCheck.vi"("error in (no error)"=w353, "enable/disable"=TRUE, "SupplyControl in"=w351) -> ("error out"=w352:errorcluster)  [unwired: 7 in, 1 out]
                      n233 = call-dynamic "LCR_Init.vi"("error in (no error)"=w352, "LCRControl in"=w356) -> ("error out"=w357:errorcluster)  [unwired: 8 in, 1 out]
                    }
                    frame #2 {
                      n234 = Wait (ms)(milliseconds to wait=u32 1000) -> ()  [unwired: 1 out]
                    }
                    frame #3 {
                      n235 = Wait (ms)(milliseconds to wait=1000) -> ()  [unwired: 1 out]
                      n236 = call-dynamic "MuxCardSwitch.vi"("Single Needle"=w362, "Probe Card Channels"=w361, "error in (no error)"=w363, "Switch to channel"=1, "Switching in"=w360) -> ("error out"=w365:errorcluster, "Switching out"=w359:refnum<class "Switching.lvclass">)  [unwired: 4 in, 1 out]
                      n237 = call-dynamic "MatrixSwitch.vi"("error in (no error)"=w365, "Action"=T5."Striptest LCR", "Switching in"=w359) -> ("error out"=w364:errorcluster)  [unwired: 6 in, 2 out]
                    }
                    frame #4 {
                      n238 = call-dynamic "LCR_TrimOC.vi"("error in (no error)"=w371, "LCRControl in"=w370) -> ("error out"=w369:errorcluster)  [unwired: 8 in, 1 out]
                    }
                    frame #5 {
                      w384 = u16 0 items=["Open", "Close"] ("Switch action")
                      n239 = call-dynamic "Supply_ZeroCheck.vi"("error in (no error)"=w376, "enable/disable"=TRUE, "SupplyControl in"=w378) -> ("error out"=w375:errorcluster)  [unwired: 7 in, 1 out]
                      n240 = call-dynamic "MatrixSwitchSingle.vi"("Switch action"=w384, "error in (no error)"=w375, "Matrix Y"=1, "Matrix X"=3, "Switching in"=w377) -> ("error out"=w380:errorcluster, "Switching out"=w381:refnum<class "Switching.lvclass">)  [unwired: 4 in, 1 out]
                      n241 = call-dynamic "MatrixSwitchSingle.vi"("Switch action"=w384, "error in (no error)"=w380, "Matrix Y"=2, "Matrix X"=4, "Switching in"=w381) -> ("error out"=w379:errorcluster, "Switching out"=w374:refnum<class "Switching.lvclass">)  [unwired: 4 in, 1 out]
                      n242 = call-dynamic "MuxCardSwitch.vi"("Single Needle"=w372, "Probe Card Channels"=w373, "error in (no error)"=w379, "Switch to channel"=-1, "Switching in"=w374) -> ()  [unwired: 4 in, 3 out]
                    }
                  }
                  n243 = local write "Bias On/Off:"(TRUE ("Bias On?")) -> ()
                }
                frame True {
                  n244 = property on="Bias On/Off:" class="Bool (strict)"("Blinking"=w390) -> ()  [unwired: 2 in, 2 out]
                  n245 = local write "Status:"("Compliance exceeded\nRUN ABORTED") -> ()
                }
              }
            }
            frame True {
            }
          }
        }
        frame #3 {
          n246 = property on="Bias On/Off:" class="Bool (strict)"() -> ("Blinking"=w392:bool)  [unwired: 2 in, 2 out]
          n247 = case shown="False" w392 {
            tunnel: w393 -> [w397 _]
            tunnel: w391 -> [w394 _]
            frame False {
              w398 = 0
              n248 = property on="Abort" class="Bool (strict)"("DisabledEnum"=w398) -> ()  [unwired: 2 in, 2 out]
              n249 = property on="Auto ReCheck" class="Bool (strict)"("DisabledEnum"=w398) -> ()  [unwired: 2 in, 2 out]
              n250 = local read "Single Needle"() -> (w396:bool)
              n251 = Or(x=w396, y=w397) -> (x .or. y?=w395:bool)
              n252 = case shown="False" w395 {
                tunnel: [w401 FALSE] -> w399
                tunnel: w394 -> [w400 _]
                frame False {
                  n253 = stacked-sequence {
                    tunnel: [_ w410] -> w401
                    tunnel: w400 -> [_ _]
                    frame #0 {
                      n254 = local write "Status:"("Reference measurement") -> ()
                      n255 = global read "QC_MeasurementSetup.vi" "Striptest Measurement Parameters"() -> (w402:T7)
                      n256 = Unbundle By Name(w402) -> ("Switching"=w403:refnum<class "Switching.lvclass">)
                      n257 = call-dynamic "MatrixSwitch.vi"("Action"=T5."Striptest SMU", "Switching in"=w403) -> ()  [unwired: 7 in, 3 out]
                    }
                    frame #1 {
                      n258 = local read "settling\ndelay [ms]"() -> (w409:i32)
                      n259 = call "CurrentCorrection.vi"("Action"=T6."Reference measurement", "settling\ndelay"=w409) -> ("Compliance exceeded?"=w410:bool, "Current Reference 100V"=→"Current Reference 100V":dbl[], "Current Reference 10V"=→"Current Reference 10V":dbl[])  [unwired: 3 in, 2 out]
                    }
                  }
                }
                frame True {
                }
              }
              n260 = case shown="False" w399 {
                frame False {
                  n261 = local write "Status:"("RUN IN PROGRESS" ("STATUS 1")) -> ()
                }
                frame True {
                  n262 = property on="Bias On/Off:" class="Bool (strict)"("Blinking"=TRUE ("Compliance?")) -> ()  [unwired: 2 in, 2 out]
                  n263 = local write "Status:"("Compliance exceeded\nRUN ABORTED") -> ()
                }
              }
            }
            frame True {
            }
          }
        }
        frame #4 {
          n264 = property on="Bias On/Off:" class="Bool (strict)"() -> ("Blinking"=w417:bool)  [unwired: 2 in, 2 out]
          n265 = case shown="False" w417 {
            tunnel: w418 -> [w428 _]
            tunnel: w416 -> [w427 _]
            tunnel: w415 -> [w426 _]
            frame False {
              n266 = Array Size(array=w428) -> (size(s)=w429:i32)
              n267 = local read "Temperature Progression"() -> (w420:T3)
              n268 = local read "probe points per region"() -> (w421:i32[])
              n269 = local read "max scale array"() -> (w424:i32[])
              n270 = local read "min scale array"() -> (w423:i32[])
              n271 = for {
                N: w429 -> [_]
                tunnel: w428 -> [w442] mode=indexing
                tunnel: w427 -> [w441] mode=indexing
                tunnel: w426 -> [w440]
                shift-right: [w434] -> _
                shift-left: 0 -> [w439]
                tunnel: w424 -> [w437] mode=indexing
                tunnel: w423 -> [w438] mode=indexing
                shift-right: [w433] -> _
                shift-left: 0 -> [w435]
                tunnel: w421 -> [w432] mode=indexing
                shift-right: [w430] -> w419
                shift-left: w420 -> [w431]
                i -> [w436]
                n272 = case shown="True" w442 {
                  tunnel: w441 -> [_ w458]
                  tunnel: w440 -> [_ _]
                  tunnel: w439 -> [w444 w459]
                  tunnel: w438 -> [_ w454]
                  tunnel: w437 -> [_ w451]
                  tunnel: w436 -> [_ w456]
                  tunnel: w435 -> [w446 w453]
                  tunnel: [w443 w452] -> w434
                  tunnel: [w446 w450] -> w433
                  tunnel: w432 -> [_ w449]
                  tunnel: w431 -> [w445 w448]
                  tunnel: [w445 w447] -> w430
                  frame False {
                    n273 = Increment(x=w444) -> (x+1=w443:i32)
                  }
                  frame True {
                    n274 = local write "Show:"(w459) -> ()
                    n275 = Unbundle By Name(w458) -> ("Region"=→"Probing Region:":string, "ProbePoints"=w455:T13)
                    n276 = while {
                      tunnel: w456 -> [w460]
                      tunnel: w455 -> [w480]
                      shift-right: [w473] -> _
                      shift-left: w454 -> [w462]
                      shift-right: [w474] -> w450
                      shift-left: w453 -> [w475]
                      tunnel: w451 -> [w472]
                      tunnel: w449 -> [_]
                      shift-right: [w470] -> w447
                      shift-left: w448 -> [w471]
                      i -> [w476]
                      stop <- w479 stop-if-true
                      n277 = Index Array(array=w480, index=w462) -> (element=w481:T14)
                      n278 = Equal To 0?(x=w475) -> (x = 0?=w482:bool)
                      n279 = Equal?(x=w462, y=w472) -> (x = y?=w461:bool)
                      n280 = case shown="True" w482 {
                        frame False {
                        }
                        frame True {
                          n281 = local read "Probe Card Channels"() -> (w1025:i32)
                          n282 = local read "total strip number"() -> (w1026:u32)
                          n283 = Divide(x=w1026, y=w1025) -> (x/y=w1024:dbl)
                          n284 = To Long Integer(number=w1024) -> (32bit integer=w1023:i32)
                          n285 = call "RunTime.vi"("no. measurements"=w1023, "Flag"=1) -> ()  [unwired: 2 in, 4 out]
                        }
                      }
                      n286 = case shown="True" w461 {
                        tunnel: w460 -> [_ w483]
                        frame False {
                        }
                        frame True {
                          n287 = stacked-sequence {
                            tunnel: w483 -> [_ w486 w492]
                            frame #0 {
                              n288 = Wait (ms)(milliseconds to wait=100) -> ()  [unwired: 1 out]
                            }
                            frame #1 {
                              n289 = Increment(x=w486) -> (x+1=w489:i32)
                              n290 = Multiply(x=w489, y=111) -> (x*y=w487:i32)
                              n291 = call "SaveJPEG.vi"("Picture No."=w487, "Test"="Striptest") -> ()  [unwired: 1 in, 2 out]
                            }
                            frame #2 {
                              n292 = local read "probe points per region"() -> (w496:i32[])
                              n293 = Index Array(array=w496, index=w492) -> (element=w493:i32)
                              n294 = local read "Probing Region:"() -> (w491:string)
                              n295 = call "SaveStriptestRecoveryFiles.vi"("Arrays format"="%016.6f", "Array Titles"="ProbeplanIndex Current PinholeFlag Capacitance Resistance", "Strip Segment"=w491, "no. of arrays"=5, "Actual array lengths"=w493, "Region #"=w492) -> ()  [unwired: 2 out]
                            }
                          }
                        }
                      }
                      n296 = Unbundle By Name(w481) -> ("CardViable?"=w467:bool)
                      n297 = property on="Bias On/Off:" class="Bool (strict)"() -> ("Blinking"=w477:bool)  [unwired: 2 in, 2 out]
                      n298 = property on="Bias On/Off:" class="Bool (strict)"() -> ("Blinking"=w469:bool)  [unwired: 2 in, 2 out]
                      n299 = local read "Abort"() -> (w465:bool)
                      n300 = Not(x=w469) -> (.not. x?=w468:bool)
                      n301 = Not(x=w465) -> (.not. x?=w464:bool)
                      n302 = Compound Arithmetic op=AND(w467, w468, w464) -> (w466:bool)
                      n303 = Build Array(w477, "Abort", w461) -> (w478:bool[])
                      n304 = Or Array Elements(Boolean array=w478) -> (logical OR=w479:bool)
                      n305 = case shown="True" w466 {
                        tunnel: w460 -> [_ w514]
                        tunnel: w480 -> [_ w513]
                        tunnel: w462 -> [w497 w508]
                        tunnel: w476 -> [_ w512]
                        tunnel: w475 -> [w500 w511]
                        tunnel: [w500 w510] -> w474
                        tunnel: [w498 w509] -> w473
                        tunnel: w471 -> [w499 w507]
                        tunnel: [w499 w506] -> w470
                        frame False {
                          n306 = Increment(x=w497) -> (x+1=w498:i32)
                        }
                        frame True {
                          n307 = global read "QC_MeasurementSetup.vi" "Striptest Measurement Parameters"() -> (w504:T7)
                          n308 = Unbundle By Name(w504) -> ("ProbeStation"=w503:refnum<class "ProbeStationControl.lvclass">, "Switching"=w505:refnum<class "Switching.lvclass">, "Temperature Readout"=w501:enum16{"Read Arduino", "Enter manually"}, "Arduino"=w502:refnum<class "ArduinoControl.lvclass">)
                          n309 = stacked-sequence {
                            tunnel: w514 -> [w528 w809 w899 w993 _]
                            tunnel: w513 -> [w517 _ _ _ _]
                            tunnel: w508 -> [w516 _ _ _ w1013]
                            tunnel: w511 -> [_ _ _ _ w1022]
                            tunnel: w512 -> [_ w808 w898 w992 w1011]
                            tunnel: [_ _ _ _ w1014] -> w510
                            tunnel: [_ _ _ _ w1021] -> w509
                            tunnel: w507 -> [_ w803 _ _ _]
                            tunnel: [_ w802 _ _ _] -> w506
                            tunnel: w505 -> [_ w806 w896 _ _]
                            tunnel: w503 -> [w515 _ _ _ _]
                            tunnel: w502 -> [_ w805 _ _ _]
                            tunnel: w501 -> [_ w804 _ _ _]
                            frame #0 {
                              w527 = u32 4 items=["Reset", "Read Array", "Read Element", "Write Element", "Write Array"] ("Action")
                              # "If probepoint label defined as Strip or Channel, use\nthat as the channel number in the data array."
                              n310 = local write "disabled channels"(i32[] []) -> ()
                              n311 = Index Array(array=w517, index=w516) -> (element=w535:T14)
                              n312 = Unbundle(w535) -> ("Label"=w531:string)  [unwired: 3 out]
                              "Probe Point:" <- w531
                              n313 = local read "Simulation?"() -> (w521:bool)
                              n314 = local read "Abort"() -> (w523:bool)
                              n315 = Format Into String(format string="Moving to %s", w531) -> (resulting string=w534:string)  [unwired: 2 in, 1 out]
                              n316 = local write "Status:"(w534) -> ()
                              n317 = local read "Probe Card Channels"() -> (w524:i32)
                              n318 = Or(x=w523, y=w521) -> (x .or. y?=w522:bool)
                              n319 = case shown="False" w522 {
                                tunnel: w528 -> [w794 _]
                                tunnel: w516 -> [w795 _]
                                tunnel: w524 -> [w796 _]
                                tunnel: w515 -> [w792 _]
                                frame False {
                                # "Move to Strip"
                                n320 = local read "Single Needle"() -> (w798:bool)
                                n321 = call "MoveToStrip.vi"("Single Needle"=w798, "Strip No."=w795, "Region"=w794, "ProbeStationControl in"=w792) -> ("Z [µm]"=w793:i32)  [unwired: 5 in, 2 out]
                                n322 = local read "Z profile"() -> (w801:i32[][])
                                n323 = Initialize Array(w793, w796, 1) -> (w799:i32[][])
                                n324 = Replace Array Subset(array=w801, new element=w799, index (row)=w795, index (col)=w794) -> (w800:i32[][])
                                n325 = local write "Z profile"(w800) -> ()
                                }
                                frame True {
                                }
                              }
                              n326 = xnode "Match Regular Expression"("input string"=w531, "regular expression"="(Strip|Channel)\\s+(\\d+)", "ignore case? (F)"=TRUE) -> ("submatch 2"=w520:string)  [unwired: 3 in, 6 out]
                              n327 = Empty String/Path?(string/path=w520) -> (empty?=w519:bool)
                              n328 = Not(x=w519) -> (.not. x?=w518:bool)
                              n329 = case shown="True" w518 {
                                tunnel: [w537 w547] -> w529
                                tunnel: w516 -> [w539 w545]
                                tunnel: w524 -> [w538 w546]
                                tunnel: w517 -> [_ w544]
                                frame False {
                                n330 = for {
                                N: w538 -> [_]
                                tunnel: w539 -> [w542]
                                tunnel: [w540] -> w537 mode=indexing
                                i -> [w543]
                                # "Actually use the probepoint\nindex"
                                n331 = Add(x=w542, y=w543) -> (x+y=w541:i32)
                                n332 = Increment(x=w541) -> (x+1=w540:i32)
                                }
                                }
                                frame True {
                                n333 = for {
                                N: w546 -> [_]
                                tunnel: [w556] -> w547 mode=indexing
                                tunnel: w545 -> [w553]
                                tunnel: w544 -> [w551]
                                i -> [w554]
                                n334 = Add(x=w553, y=w554) -> (x+y=w552:i32)
                                n335 = Index Array(array=w551, index=w552) -> (element=w550:T14)
                                n336 = Unbundle By Name(w550) -> ("Label"=w549:string)
                                n337 = xnode "Match Regular Expression"("input string"=w549, "regular expression"="(Strip|Channel)\\s+(\\d+)") -> ("submatch 2"=w548:string)  [unwired: 4 in, 6 out]
                                n338 = Scan From String(format string="%d", input string=w548) -> (output 1=w556:i32)  [unwired: 3 in, 3 out]
                                }
                                }
                              }
                              n339 = To Double Precision Float(number=w529) -> (double precision float=w525:dbl[])
                              n340 = call "MultiRegionData.vi"("Action"=w527, "Array No."=0 ("Array Size / Index"), "Array Size / Index"=w516, "Array IN"=w525, "Region index"=w528) -> ()  [unwired: 1 in, 2 out]
                            }
                            frame #1 {
                              # "Pinholes"
                              n341 = local read "Simulation?"() -> (w807:bool)
                              n342 = stacked-sequence {
                                tunnel: w807 -> [w825 w846]
                                tunnel: w809 -> [_ w848]
                                tunnel: w808 -> [_ w847]
                                tunnel: w806 -> [w824 _]
                                tunnel: w805 -> [w822 _]
                                tunnel: w804 -> [w823 _]
                                tunnel: w803 -> [w816 _]
                                tunnel: [w814 _] -> w802
                                frame #0 {
                                n343 = Unbundle By Name(w816) -> ("Time Array"=w818:string[], "Temperature Array [°C]"=w813:dbl[], "Humidity Array [RH %]"=w812:dbl[])
                                n344 = case shown="\"Read Arduino\", Default" w823 {
                                tunnel: w822 -> [w833 _]
                                tunnel: [w832 _] -> w821
                                tunnel: w813 -> [w828 w837]
                                tunnel: w812 -> [w829 w839]
                                tunnel: [w827 w836] -> w811
                                tunnel: [w826 w835] -> w810
                                frame "Read Arduino", Default {
                                n345 = call "ArduinoRead.vi"("Arduino function"=enum16{"T/RH", "Interlock", "Edgesense"}."T/RH", "ArduinoControl in"=w833) -> ("error out"=w832:errorcluster, "rel. Humidity [%]"=w830:dbl, "Temperature [°C]"=w831:dbl)  [unwired: 4 in, 3 out]
                                n346 = Build Array (concatenate)(w828, w831) -> (w827:dbl[])
                                n347 = Build Array (concatenate)(w829, w830) -> (w826:dbl[])
                                }
                                frame "Enter manually" {
                                n348 = Index Array(array=w837, index=0) -> (element=w838:dbl)
                                n349 = Index Array(array=w839, index=0) -> (element=w840:dbl)
                                n350 = Build Array (concatenate)(w837, w838) -> (w836:dbl[])
                                n351 = Build Array (concatenate)(w839, w840) -> (w835:dbl[])
                                }
                                }
                                n352 = call "RunTime.vi"("Probing done - new estimation"=FALSE, "Flag"=0) -> ("Time so far"=w817:string)  [unwired: 2 in, 3 out]
                                n353 = Build Array (concatenate)(w818, w817) -> (w815:string[])
                                n354 = case shown="False" w825 {
                                tunnel: w824 -> [w845 _]
                                tunnel: w821 -> [w844 _]
                                frame False {
                                n355 = call-dynamic "MatrixSwitch.vi"("error in (no error)"=w844, "Action"=T5."Striptest SMU", "Switching in"=w845) -> ()  [unwired: 6 in, 3 out]
                                }
                                frame True {
                                }
                                }
                                n356 = Bundle By Name(cluster=w816, "Time Array"=w815, "Temperature Array [°C]"=w811, "Humidity Array [RH %]"=w810) -> (w814:T3)
                                }
                                frame #1 {
                                n357 = local read "Abort"() -> (w849:bool)
                                n358 = case shown="False" w849 {
                                tunnel: w848 -> [w859 _]
                                tunnel: w847 -> [w858 _]
                                tunnel: w846 -> [w850 _]
                                frame False {
                                w855 = u32 4 items=["Reset", "Read Array", "Read Element", "Write Element", "Write Array"] ("Action")
                                w856 = u32 4 items=["Reset", "Read Array", "Read Element", "Write Element", "Write Array"] ("Action")
                                n359 = case shown="True" w850 {
                                tunnel: [w871 w884] -> w851
                                tunnel: [w868 w883] -> w857
                                frame False {
                                n360 = local read "Thresholds:"() -> (w870:T2)
                                n361 = Unbundle By Name(w870) -> ("Current [nA]"=w869:dbl)
                                n362 = case shown="False" "Rolling\nCurrent Readout" {
                                tunnel: [w876 w878] -> w871
                                tunnel: w869 -> [w872 w881]
                                tunnel: [w875 w880] -> w868
                                tunnel: [w874 w879] -> w867
                                tunnel: "settling\ndelay [ms]" -> [w873 w877]
                                frame False {
                                n363 = call "Pinholes.vi"("Current Threshold [nA]"=w872, "settling\ndelay"=w873) -> ("excluded channels"=w874:i32[], "Current [nA]"=w876:dbl[], "Flag"=w875:i32[])  [unwired: 3 in]
                                }
                                frame True {
                                n364 = call "PinholesRolling.vi"("Current Threshold [nA]"=w881, "settling\ndelay"=w877) -> ("excluded channels"=w879:i32[], "Current [nA]"=w878:dbl[], "Flag"=w880:i32[])  [unwired: 3 in]
                                }
                                }
                                "disabled channels" <- w867
                                }
                                frame True {
                                n365 = local read "Probe Card Channels"() -> (w882:i32)
                                n366 = for {
                                N: w882 -> [_]
                                tunnel: [w886] -> w884 mode=indexing
                                tunnel: [w885] -> w883 mode=indexing
                                # "Simulate"
                                n367 = Random Number (0-1)() -> (number: 0 to 1=w889:dbl)
                                n368 = Greater?(x=w889, y=0.95) -> (0:w890:bool)
                                n369 = case shown="False" w890 {
                                tunnel: [w894 5000.0] -> w886
                                tunnel: w889 -> [w894 _]
                                frame False {
                                }
                                frame True {
                                }
                                }
                                n370 = Greater?(x=w886, y=50.0) -> (0:w887:bool)
                                n371 = case shown="False" w887 {
                                tunnel: [0 1] -> w885
                                frame False {
                                }
                                frame True {
                                }
                                }
                                }
                                }
                                }
                                n372 = Get Date/Time String(want seconds? (F)=TRUE) -> (time string=→"Last Probe at:":string)  [unwired: 2 in, 1 out]
                                n373 = local write "Status:"("Measuring Ipinhole") -> ()
                                n374 = To Double Precision Float(number=w857) -> (double precision float=w854:dbl[])
                                n375 = Index Array(array=w851, index=0) -> (element=→"Current [nA]:":dbl)
                                n376 = call "MultiRegionData.vi"("Action"=w855, "Array No."=1, "Array Size / Index"=w858, "Array IN"=w851, "Region index"=w859) -> ()  [unwired: 1 in, 2 out]
                                n377 = call "MultiRegionData.vi"("Action"=w856, "Array No."=2, "Array Size / Index"=w858, "Array IN"=w854, "Region index"=w859) -> ()  [unwired: 1 in, 2 out]
                                }
                                frame True {
                                }
                                }
                                }
                              }
                            }
                            frame #2 {
                              # "Capacitance and Resistance"
                              n378 = local read "Simulation?"() -> (w897:bool)
                              n379 = stacked-sequence {
                                seq-local: [_ _ w911 _] -> [_ _ _ w972]
                                tunnel: w899 -> [_ _ w921 _]
                                tunnel: w898 -> [_ _ w920 _]
                                tunnel: w897 -> [w901 w905 w910 w971]
                                tunnel: w896 -> [w900 w904 w909 w970]
                                frame #0 {
                                n380 = case shown="False" w901 {
                                tunnel: w900 -> [w902 _]
                                frame False {
                                n381 = call-dynamic "MatrixSwitch.vi"("Action"=T5."Ground", "Switching in"=w902) -> ()  [unwired: 7 in, 3 out]
                                }
                                frame True {
                                }
                                }
                                }
                                frame #1 {
                                n382 = case shown="False" w905 {
                                tunnel: w904 -> [w907 _]
                                frame False {
                                n383 = call-dynamic "MatrixSwitch.vi"("Action"=T5."Striptest LCR", "Switching in"=w907) -> ()  [unwired: 7 in, 3 out]
                                }
                                frame True {
                                }
                                }
                                n384 = local write "Status:"("Measuring capacitance..." ("STATUS 1")) -> ()
                                }
                                frame #2 {
                                w914 = 0
                                w918 = u32 4 items=["Reset", "Read Array", "Read Element", "Write Element", "Write Array"] ("Action")
                                w919 = u32 4 items=["Reset", "Read Array", "Read Element", "Write Element", "Write Array"] ("Action")
                                n385 = local read "Probe Card Channels"() -> (w911:i32)
                                n386 = local read "disabled channels"() -> (w913:i32[])
                                n387 = for {
                                N: w911 -> [_]
                                tunnel: [w930] -> w912 mode=indexing
                                tunnel: [w929] -> w915 mode=indexing
                                tunnel: w913 -> [w926]
                                tunnel: w911 -> [w928]
                                tunnel: w910 -> [w925]
                                tunnel: w909 -> [w924]
                                i -> [w927]
                                n388 = case shown="False" w925 {
                                tunnel: [w939 w961] -> w930
                                tunnel: [w938 w960] -> w929
                                tunnel: w928 -> [w935 _]
                                tunnel: w927 -> [w933 _]
                                tunnel: w926 -> [w934 _]
                                tunnel: w924 -> [w931 _]
                                frame False {
                                n389 = Increment(x=w933) -> (x+1=w932:i32)
                                n390 = Search 1D Array(1D array=w934, element=w932) -> (index of element=w937:i32)  [unwired: 1 in]
                                n391 = Less Than 0?(x=w937) -> (x < 0?=w936:bool)
                                n392 = case shown="True" w936 {
                                tunnel: [w942 w948] -> w939
                                tunnel: [w940 w947] -> w938
                                tunnel: w935 -> [_ w946]
                                tunnel: w932 -> [_ w945]
                                tunnel: w934 -> [_ w944]
                                tunnel: w931 -> [_ w943]
                                frame False {
                                w942 = -1.0
                                n393 = Divide(x=w942, y=1000000.0) -> (x/y=w940:dbl)
                                }
                                frame True {
                                n394 = stacked-sequence {
                                tunnel: w946 -> [w951 _ _]
                                tunnel: w945 -> [w953 _ _]
                                tunnel: w944 -> [w952 _ _]
                                tunnel: [_ _ w959] -> w948
                                tunnel: [_ _ w958] -> w947
                                tunnel: w943 -> [w950 _ _]
                                frame #0 {
                                n395 = local read "Single Needle"() -> (w949:bool)
                                n396 = call-dynamic "MuxCardSwitch.vi"("Single Needle"=w949, "Probe Card Channels"=w951, "disabled channels"=w952, "Switch to channel"=w953, "Switching in"=w950) -> ()  [unwired: 4 in, 3 out]
                                }
                                frame #1 {
                                n397 = local read "settling\ndelay [ms]"() -> (w954:i32)
                                n398 = Wait (ms)(milliseconds to wait=w954) -> ()  [unwired: 1 out]
                                }
                                frame #2 {
                                n399 = global read "QC_MeasurementSetup.vi" "Striptest Measurement Parameters"() -> (w957:T7)
                                n400 = Unbundle By Name(w957) -> ("LCR"=w956:refnum<class "LCRControl.lvclass">, "AC frequency [Hz]"=w955:i32)
                                n401 = call-dynamic "LCR_Readout.vi"("Frequency in Hz"=w955, "LCRControl in"=w956) -> ("Resistance in Ohm"=w958:dbl, "Capacitance in pF"=w959:dbl)  [unwired: 6 in, 2 out]
                                }
                                }
                                }
                                }
                                }
                                frame True {
                                n402 = Random Number (0-1)() -> (number: 0 to 1=w965:dbl)
                                n403 = Random Number (0-1)() -> (number: 0 to 1=w969:dbl)
                                n404 = Multiply(x=w969, y=18.0) -> (x*y=w967:dbl)
                                n405 = Multiply(x=w965, y=0.6) -> (x*y=w962:dbl)
                                n406 = Add(x=w967, y=64.0) -> (x+y=w961:dbl)
                                n407 = Add(x=1.5 ("Resistance"), y=w962) -> (x+y=w960:dbl)
                                }
                                }
                                }
                                n408 = Index Array(array=w915, index=w914) -> (element=→"Reistance [MW]:":dbl)
                                n409 = Index Array(array=w912, index=w914) -> (element=→"Capacitance [pF]:":dbl)
                                n410 = call "MultiRegionData.vi"("Action"=w919, "Array No."=3, "Array Size / Index"=w920, "Array IN"=w912, "Region index"=w921) -> ()  [unwired: 1 in, 2 out]
                                n411 = call "MultiRegionData.vi"("Action"=w918, "Array No."=4, "Array Size / Index"=w920, "Array IN"=w915, "Region index"=w921) -> ()  [unwired: 1 in, 2 out]
                                }
                                frame #3 {
                                n412 = case shown="False" w971 {
                                tunnel: w972 -> [w975 _]
                                tunnel: w970 -> [w973 _]
                                frame False {
                                n413 = local read "Single Needle"() -> (w974:bool)
                                n414 = call-dynamic "MuxCardSwitch.vi"("Single Needle"=w974, "Probe Card Channels"=w975, "Switch to channel"=-1, "Switching in"=w973) -> ()  [unwired: 5 in, 3 out]
                                }
                                frame True {
                                }
                                }
                                }
                              }
                            }
                            frame #3 {
                              # "If selected region is CURRENT region being probed,\nuse number probed so far\notherwise total number of probepoints in this region"
                              n415 = local read "Region Indices"() -> (w995:i32[])
                              n416 = Index Array(array=w995, index="Show:") -> (element=w991:i32)
                              n417 = Equal?(x=w991, y=w993) -> (x = y?=w994:bool)
                              n418 = case shown="True" w994 {
                                tunnel: w992 -> [_ w1007]
                                tunnel: [w1003 w1006] -> w990
                                tunnel: w991 -> [w1002 _]
                                frame False {
                                n419 = local read "probe points per region"() -> (w1004:i32[])
                                n420 = Index Array(array=w1004, index=w1002) -> (element=w1003:i32)
                                }
                                frame True {
                                n421 = local read "Probe Card Channels"() -> (w1005:i32)
                                n422 = Add(x=w1005, y=w1007) -> (x+y=w1006:i32)
                                }
                              }
                              n423 = local read "max scale array"() -> (w987:i32[])
                              n424 = local read "min scale array"() -> (w989:i32[])
                              n425 = local read "Thresholds:"() -> (w1001:T2)
                              n426 = Index Array(array=w987, index="Show:") -> (element=w984:i32)
                              n427 = Index Array(array=w989, index="Show:") -> (element=w986:i32)
                              n428 = call "DisplayStriptestData.vi"("min scale array"=w989, "max scale array"=w987, "# probed"=w990, "Display Stats?"=TRUE, "Thresholds"=w1001, "Region"=w991) -> ("Defects"=→"Defects":i32[][], "Resistance [MW]"=→"Resistance [MW]":cluster{u32, i32, "Array OUT":dbl[]}, "Capacitance [pF]"=→"Capacitance [pF]":cluster{u32, i32, "Array OUT":dbl[]}, "Current [nA]"=→"Current [nA]":cluster{u32, i32, "Array OUT":dbl[]}, "Strip Quality Data"=w997:T15)
                              n429 = Increment(x=w984) -> (x+1=w983:i32)
                              n430 = Increment(x=w986) -> (x+1=w985:i32)
                              n431 = property on="Capacitance [pF]" class="WFGraph (strict)"("XScale.Maximum"=w983) -> ()  [unwired: 2 in, 2 out]
                              n432 = property on="Resistance [MW]" class="WFGraph (strict)"("XScale.Maximum"=w983) -> ()  [unwired: 2 in, 2 out]
                              n433 = property on="Current [nA]" class="WFGraph (strict)"("XScale.Maximum"=w983) -> ()  [unwired: 2 in, 2 out]
                              n434 = property on="Capacitance [pF]" class="WFGraph (strict)"("XScale.Minimum"=w985) -> ()  [unwired: 2 in, 2 out]
                              n435 = property on="Resistance [MW]" class="WFGraph (strict)"("XScale.Minimum"=w985) -> ()  [unwired: 2 in, 2 out]
                              n436 = property on="Current [nA]" class="WFGraph (strict)"("XScale.Minimum"=w985) -> ()  [unwired: 2 in, 2 out]
                              n437 = property on="Defects" class="IntGraph (strict)"("XScale.Minimum"=w985) -> ()  [unwired: 2 in, 2 out]
                              n438 = Increment(x=w983) -> (x+1=w982:i32)
                              n439 = property on="Defects" class="IntGraph (strict)"("XScale.Maximum"=w982) -> ()  [unwired: 2 in, 2 out]
                              n440 = Unbundle By Name(w997) -> ("pass Rate in %"=→"% OK:":dbl, "Bad channel list"=→"Bad Strip List":i32[], "No of bad strips"=w980:i32, "Number of defects per category"=→"defect type array":i32[])
                              n441 = local write "# total defects:"(w980) -> ()
                            }
                            frame #4 {
                              # "save image if required"
                              n442 = call "RunTime.vi"("Probing done - new estimation"=TRUE, "Flag"=0) -> ("Estimated Completion Time"=w1018:string, "Time so far"=→"Run Duration:":string)  [unwired: 2 in, 2 out]
                              n443 = Scan From String(format string="%s %s", input string=w1018) -> (output 2=→"Estimated Completion:":string)  [unwired: 5 in, 3 out]
                              n444 = local read "Probe Card Channels"() -> (w1012:i32)
                              n445 = Quotient & Remainder(x=w1011, y=w1012) -> (floor(x/y)=w1010:i32)  [unwired: 1 out]
                              n446 = Add(x=w1012, y=w1022) -> (x+y=w1014:i32)
                              n447 = Increment(x=w1010) -> (x+1=w1009:i32)
                              n448 = local write "# probed"(w1014) -> ()
                              n449 = call "SaveJPEG.vi"("Picture No."=w1009, "Test"="Striptest") -> ()  [unwired: 1 in, 2 out]
                              n450 = Increment(x=w1013) -> (x+1=w1021:i32)
                            }
                          }
                        }
                      }
                    }
                    n451 = Increment(x=w459) -> (x+1=w452:i32)
                  }
                }
              }
              n452 = local write "Temperature Progression"(w419) -> ()
            }
            frame True {
            }
          }
        }
        frame #5 {
          # "Ramp down volts now"
          n453 = case shown="False" w1029 {
            tunnel: w1028 -> [w1050 _]
            frame False {
              w1055 = "0"
              n454 = property on="Abort" class="Bool (strict)"("DisabledEnum"=2) -> ()  [unwired: 2 in, 2 out]
              n455 = local read "# probed"() -> (w1048:i32)
              n456 = call-dynamic "Prober_ChuckUpDown.vi"("Direction"=enum16{"up", "down"}."down", "ProbeStationControl in"=w1050) -> ("error out"=w1052:errorcluster, "ProbeStationControl out"=w1051:refnum<class "ProbeStationControl.lvclass">)  [unwired: 7 in, 1 out]
              n457 = call "SaveJPEG.vi"("Picture No."=w1048, "Test"="Striptest") -> ()  [unwired: 1 in, 2 out]
              n458 = call-dynamic "Prober_MoveToXYZTheta.vi"("Theta location [mdeg]"="none", "ProbeStationControl in"=w1051, "error in (no error)"=w1052, "Z location [µm]"="down", "Y location [µm]"=w1055, "X location [µm]"=w1055) -> ()  [unwired: 3 in, 3 out]
            }
            frame True {
            }
          }
          n459 = local read "Abort"() -> (w1041:bool)
          n460 = property on="Bias On/Off:" class="Bool (strict)"() -> ("Blinking"=w1040:bool)  [unwired: 2 in, 2 out]
          n461 = Not Or(1:w1041, 2:w1040) -> (0:w1039:bool)
          n462 = Build Array(w1039, w1040, w1041) -> (w1042:bool[])
          n463 = Search 1D Array(1D array=w1042, element=TRUE) -> (index of element=w1044:i32)  [unwired: 1 in]
          n464 = Increment(x=w1044) -> (x+1=w1030:i32)
          n465 = Pick Line(multi-line string=" null\n Run ended normally.\n Compliance exceeded. \n Run aborted early.", line index=w1030) -> (output string=w1031:string)  [unwired: 1 in]
          n466 = global read "QC_RunInformation.vi" "Run info"() -> (w1033:T8)
          n467 = Bundle By Name(cluster=w1033, "End of Run comment:"=w1031) -> (w1032:T8)
          n468 = global write "QC_RunInformation.vi" "Run info"(w1032) -> ()
          n469 = Concatenate Strings(" End of Run.", "\r\n", w1031) -> (w1034:string)
          n470 = Concatenate Strings(w1031, "\r\n", "RAMPING DOWN VOLTS") -> (w1037:string)
          n471 = stacked-sequence {
            tunnel: w1037 -> [w1057 _ _ _]
            tunnel: w1034 -> [_ _ w1061 _]
            frame #0 {
              n472 = local write "Status:"(w1057) -> ()
            }
            frame #1 {
              n473 = local read "Simulation?"() -> (w1058:bool)
              n474 = case shown="False" w1058 {
                frame False {
                  n475 = global read "QC_MeasurementSetup.vi" "Striptest Measurement Parameters"() -> (w1060:T7)
                  n476 = Unbundle By Name(w1060) -> ("SMU"=w1059:refnum<class "SupplyControl.lvclass">)
                  n477 = call-dynamic "Supply_Stby.vi"("SupplyControl in"=w1059) -> ()  [unwired: 9 in, 2 out]
                }
                frame True {
                }
              }
            }
            frame #2 {
              n478 = local write "Status:"(w1061) -> ()
            }
            frame #3 {
              w1064 = 0
              n479 = property on="Save Data" class="Bool (strict)"("DisabledEnum"=w1064) -> ()  [unwired: 2 in, 2 out]
              n480 = property on="Quit w/o saving" class="Bool (strict)"("DisabledEnum"=w1064) -> ()  [unwired: 2 in, 2 out]
              n481 = property on="ReCheck" class="Bool"("DisabledEnum"=w1064) -> ()  [unwired: 2 in, 2 out]
              n482 = property on="Auto ReCheck" class="Bool (strict)"("DisabledEnum"=1) -> ()  [unwired: 2 in, 2 out]
              n483 = local write "Status:"("Run finished. \nSave data?" ("STATUS 1")) -> ()
            }
          }
        }
        frame #6 {
          w1075 = ""
          n484 = stacked-sequence {
            tunnel: [w1097 _ _ _] -> w1093
            tunnel: [w1096 _ _ _] -> w1092
            tunnel: w1086 -> [_ w1200 w1215 _]
            tunnel: w1085 -> [w1095 _ _ _]
            frame #0 {
              # "Loop and await decision on whether to save or junk data"
              n485 = local read "Show:"() -> (w1098:u16)
              n486 = while {
                shift-right: [w1106] -> _
                shift-left: w1098 -> [w1107]
                tunnel: ["Save Data"] -> w1096
                tunnel: ["Quit w/o saving"] -> w1097
                tunnel: w1095 -> [w1099]
                stop <- w1110 stop-if-true
                # "display data if selected region changes"
                n487 = Wait (ms)(milliseconds to wait=u32 200) -> ()  [unwired: 1 out]
                n488 = local read "Show:"() -> (w1108:u16)
                n489 = Not Equal?(x=w1108, y=w1107) -> (x != y?=w1109:bool)
                n490 = Or(x="ReCheck", y="Auto ReCheck") -> (x .or. y?=w1101:bool)
                n491 = case shown="True" w1101 {
                  tunnel: "Auto ReCheck" -> [_ w1112]
                  tunnel: w1099 -> [_ w1111]
                  frame False {
                  }
                  frame True {
                    n492 = case shown="True" w1112 {
                      tunnel: w1111 -> [_ w1142]
                      frame False {
                        n493 = local read "probe points per region"() -> (w1119:i32[])
                        n494 = local read "Region Indices"() -> (w1120:i32[])
                        n495 = local read "Show:"() -> (w1118:u16)
                        n496 = Index Array(array=w1120, index=w1118) -> (element=w1117:i32)
                        n497 = Index Array(array=w1119, index=w1118) -> (element=w1116:i32)
                        n498 = flat-sequence {
                          tunnel: w1117 -> [w1121]
                          tunnel: w1116 -> [w1125]
                          tunnel: [w1121] -> w1115
                          tunnel: [w1125] -> w1114
                          tunnel: [w1124] -> w1113
                          tunnel: w1115 -> [w1141]
                          tunnel: w1114 -> [w1138]
                          tunnel: w1113 -> [w1127]
                          frame #0 {
                            n499 = local read "Probe Card Channels"() -> (w1122:i32)
                            n500 = local read "Auto ReCheck"() -> (w1123:bool)
                            n501 = local read "Thresholds:"() -> (w1126:T2)
                            n502 = call "ReCheckStrips.vi"("Probe Card Channels"=w1122, "Auto Re-Check"=w1123, "Thresholds"=w1126, "region in"=w1121, "Number of strips probed"=w1125) -> ("Thresholds copy"=w1124:T16)  [unwired: 6 in]
                            n503 = local write "Thresholds:"(w1124) -> ()
                          }
                          frame #1 {
                            n504 = local read "max scale array"() -> (w1140:i32[])
                            n505 = local read "min scale array"() -> (w1139:i32[])
                            n506 = call "DisplayStriptestData.vi"("min scale array"=w1139, "max scale array"=w1140, "# probed"=w1138, "Display Stats?"=TRUE, "Thresholds"=w1127, "Region"=w1141) -> ("Defects"=w1133:i32[][], "Resistance [MW]"=w1134:cluster{u32, i32, "Array OUT":dbl[]}, "Capacitance [pF]"=w1136:cluster{u32, i32, "Array OUT":dbl[]}, "Current [nA]"=w1135:cluster{u32, i32, "Array OUT":dbl[]}, "Strip Quality Data"=w1132:T15)
                            n507 = Unbundle By Name(w1132) -> ("pass Rate in %"=w1131:dbl, "Bad channel list"=w1130:i32[], "No of bad strips"=w1129:i32, "Defect description list"=w1128:i32[])
                            n508 = local write "Current [nA]"(w1135) -> ()
                            n509 = local write "Capacitance [pF]"(w1136) -> ()
                            n510 = local write "Resistance [MW]"(w1134) -> ()
                            n511 = local write "Defects"(w1133) -> ()
                            n512 = local write "% OK:"(w1131) -> ()
                            n513 = local write "Bad Strip List"(w1130) -> ()
                            n514 = local write "# total defects:"(w1129) -> ()
                            n515 = local write "defect type array"(w1128) -> ()
                          }
                        }
                      }
                      frame True {
                        n516 = flat-sequence {
                          tunnel: w1142 -> [w1143]
                          frame #0 {
                            n517 = local read "Region Indices"() -> (w1144:i32[])
                            n518 = Array Size(array=w1144) -> (size(s)=w1145:i32)
                            n519 = for {
                              N: w1145 -> [_]
                              tunnel: w1144 -> [w1147] mode=indexing
                              tunnel: w1143 -> [w1146] mode=indexing
                              n520 = case shown="True" w1146 {
                                tunnel: w1147 -> [_ w1151]
                                frame False {
                                }
                                frame True {
                                n521 = local read "probe points per region"() -> (w1153:i32[])
                                n522 = Index Array(array=w1153, index=w1151) -> (element=w1152:i32)
                                n523 = flat-sequence {
                                tunnel: w1151 -> [w1158]
                                tunnel: w1152 -> [w1157]
                                tunnel: [w1158] -> w1150
                                tunnel: [w1157] -> w1149
                                tunnel: [w1156] -> w1148
                                tunnel: w1150 -> [w1174]
                                tunnel: w1149 -> [w1171]
                                tunnel: w1148 -> [w1160]
                                frame #0 {
                                n524 = local read "Probe Card Channels"() -> (w1154:i32)
                                n525 = local read "Auto ReCheck"() -> (w1155:bool)
                                n526 = local read "Thresholds:"() -> (w1159:T2)
                                n527 = call "ReCheckStrips.vi"("Probe Card Channels"=w1154, "Auto Re-Check"=w1155, "Thresholds"=w1159, "region in"=w1158, "Number of strips probed"=w1157) -> ("Thresholds copy"=w1156:T16)  [unwired: 6 in]
                                n528 = local write "Thresholds:"(w1156) -> ()
                                }
                                frame #1 {
                                n529 = local read "max scale array"() -> (w1173:i32[])
                                n530 = local read "min scale array"() -> (w1172:i32[])
                                n531 = call "DisplayStriptestData.vi"("min scale array"=w1172, "max scale array"=w1173, "# probed"=w1171, "Display Stats?"=TRUE, "Thresholds"=w1160, "Region"=w1174) -> ("Defects"=w1166:i32[][], "Resistance [MW]"=w1167:cluster{u32, i32, "Array OUT":dbl[]}, "Capacitance [pF]"=w1169:cluster{u32, i32, "Array OUT":dbl[]}, "Current [nA]"=w1168:cluster{u32, i32, "Array OUT":dbl[]}, "Strip Quality Data"=w1165:T15)
                                n532 = Unbundle By Name(w1165) -> ("pass Rate in %"=w1164:dbl, "Bad channel list"=w1163:i32[], "No of bad strips"=w1162:i32, "Number of defects per category"=w1161:i32[])
                                n533 = local write "Current [nA]"(w1168) -> ()
                                n534 = local write "Capacitance [pF]"(w1169) -> ()
                                n535 = local write "Resistance [MW]"(w1167) -> ()
                                n536 = local write "Defects"(w1166) -> ()
                                n537 = local write "% OK:"(w1164) -> ()
                                n538 = local write "Bad Strip List"(w1163) -> ()
                                n539 = local write "# total defects:"(w1162) -> ()
                                n540 = local write "defect type array"(w1161) -> ()
                                }
                                }
                                }
                              }
                            }
                          }
                          frame #1 {
                            n541 = local write "Auto ReCheck"(FALSE) -> ()
                          }
                        }
                      }
                    }
                  }
                }
                n542 = case shown="True" w1109 {
                  tunnel: w1108 -> [w1176 w1183]
                  tunnel: [w1176 w1183] -> w1106
                  frame False {
                  }
                  frame True {
                    n543 = local read "probe points per region"() -> (w1193:i32[])
                    n544 = local read "Region Indices"() -> (w1184:i32[])
                    n545 = local read "max scale array"() -> (w1194:i32[])
                    n546 = local read "min scale array"() -> (w1195:i32[])
                    n547 = local read "Thresholds:"() -> (w1198:T2)
                    n548 = Index Array(array=w1184, index=w1183) -> (element=w1182:i32)
                    n549 = Index Array(array=w1193, index=w1183) -> (element=w1199:i32)
                    n550 = Index Array(array=w1194, index=w1183) -> (element=w1181:i32)
                    n551 = Index Array(array=w1195, index=w1183) -> (element=w1180:i32)
                    n552 = call "DisplayStriptestData.vi"("min scale array"=w1195, "max scale array"=w1194, "# probed"=w1199, "Display Stats?"=TRUE, "Thresholds"=w1198, "Region"=w1182) -> ("Defects"=w1196:i32[][], "Resistance [MW]"=w1190:cluster{u32, i32, "Array OUT":dbl[]}, "Capacitance [pF]"=w1191:cluster{u32, i32, "Array OUT":dbl[]}, "Current [nA]"=w1192:cluster{u32, i32, "Array OUT":dbl[]}, "Strip Quality Data"=w1197:T15)
                    n553 = Increment(x=w1181) -> (x+1=w1178:i32)
                    n554 = Increment(x=w1180) -> (x+1=w1179:i32)
                    n555 = property on="Resistance [MW]" class="WFGraph (strict)"("XScale.Minimum"=w1179) -> ()  [unwired: 2 in, 2 out]
                    n556 = property on="Resistance [MW]" class="WFGraph (strict)"("XScale.Maximum"=w1178) -> ()  [unwired: 2 in, 2 out]
                    n557 = property on="Current [nA]" class="WFGraph (strict)"("XScale.Maximum"=w1178) -> ()  [unwired: 2 in, 2 out]
                    n558 = Unbundle By Name(w1197) -> ("pass Rate in %"=w1187:dbl, "Bad channel list"=w1185:i32[], "No of bad strips"=w1188:i32, "Number of defects per category"=w1186:i32[])
                    n559 = property on="Capacitance [pF]" class="WFGraph (strict)"("XScale.Minimum"=w1179) -> ()  [unwired: 2 in, 2 out]
                    n560 = property on="Defects" class="IntGraph (strict)"("XScale.Minimum"=w1179) -> ()  [unwired: 2 in, 2 out]
                    n561 = local write "Current [nA]"(w1192) -> ()
                    n562 = local write "Capacitance [pF]"(w1191) -> ()
                    n563 = property on="Current [nA]" class="WFGraph (strict)"("XScale.Minimum"=w1179) -> ()  [unwired: 2 in, 2 out]
                    n564 = local write "Resistance [MW]"(w1190) -> ()
                    n565 = local write "Defects"(w1196) -> ()
                    n566 = property on="Capacitance [pF]" class="WFGraph (strict)"("XScale.Maximum"=w1178) -> ()  [unwired: 2 in, 2 out]
                    n567 = Increment(x=w1178) -> (x+1=w1177:i32)
                    n568 = property on="Defects" class="IntGraph (strict)"("XScale.Maximum"=w1177) -> ()  [unwired: 2 in, 2 out]
                    n569 = local write "% OK:"(w1187) -> ()
                    n570 = local write "Bad Strip List"(w1185) -> ()
                    n571 = local write "# total defects:"(w1188) -> ()
                    n572 = local write "defect type array"(w1186) -> ()
                  }
                }
                n573 = Or(x="Save Data", y="Quit w/o saving") -> (x .or. y?=w1110:bool)
              }
              n574 = local write "Save Data"("Auto quit &\nswitch off bias") -> ()
            }
            frame #1 {
              n575 = case shown="False" w1200 {
                frame False {
                  # "supply to standby"
                  n576 = global read "QC_MeasurementSetup.vi" "Striptest Measurement Parameters"() -> (w1212:T7)
                  n577 = Unbundle By Name(w1212) -> ("Bias Supply"=w1201:refnum<class "SupplyControl.lvclass">, "Switching"=w1211:refnum<class "Switching.lvclass">)
                  n578 = local read "Current Bias Voltage [V]"() -> (w1205:dbl)
                  n579 = call-dynamic "MatrixSwitch.vi"("Action"=T5."Reset", "Switching in"=w1211) -> ("error out"=w1210:errorcluster)  [unwired: 7 in, 2 out]
                  n580 = call "SupplyRamp.vi"("error in"=w1210, "Requested Voltage"=0.0, "Step Size"=10.0, "Step Delay"=1000, "Supply IN"=w1201, "Starting Voltage"=w1205) -> ("error out"=w1208:errorcluster, "Supply OUT"=w1207:refnum<class "SupplyControl.lvclass">, "Current Voltage"=w1206:dbl)  [unwired: 2 in, 1 out]
                  n581 = local write "Current Bias Voltage [V]"(w1206) -> ()
                  n582 = call-dynamic "Supply_Stby.vi"("error in (no error)"=w1208, "SupplyControl in"=w1207) -> ()  [unwired: 8 in, 2 out]
                }
                frame True {
                }
              }
            }
            frame #2 {
              n583 = case shown="False" w1215 {
                frame False {
                  n584 = global read "QC_MeasurementSetup.vi" "Striptest Measurement Parameters"() -> (w1217:T7)
                  n585 = Unbundle By Name(w1217) -> ("Arduino"=w1222:refnum<class "ArduinoControl.lvclass">)
                  n586 = local read "Temperature Progression"() -> (w1227:T3)
                  n587 = call "ArduinoRead.vi"("Arduino function"=enum16{"T/RH", "Interlock", "Edgesense"}."T/RH", "ArduinoControl in"=w1222) -> ("error out"=w1228:errorcluster, "Temperature [°C]"=w1219:dbl, "ArduinoControl out"=w1229:refnum<class "ArduinoControl.lvclass">)  [unwired: 4 in, 3 out]
                  "Last Temperature [°C]" <- w1219
                  n588 = call "ArduinoClose.vi"("error in (no error)"=w1228, "ArduinoControl in"=w1229) -> ()  [unwired: 8 in, 2 out]
                  n589 = local read "Run Duration:"() -> (w1224:string)
                  n590 = Unbundle(w1227) -> ("Time Array"=w1225:string[], "Temperature Array [°C]"=w1220:dbl[])  [unwired: 1 out]
                  n591 = Build Array (concatenate)(w1225, w1224) -> (w1223:string[])
                  n592 = Build Array (concatenate)(w1220, w1219) -> (w1218:dbl[])
                  n593 = Bundle(cluster=w1227, "Time Array"=w1223, "Temperature Array [°C]"=w1218) -> (w1226:T3)  [unwired: 1 in]
                  n594 = local write "Temperature Progression"(w1226) -> ()
                }
                frame True {
                }
              }
              n595 = local read "# probed"() -> (w1214:i32)
              n596 = call "SaveJPEG.vi"("Picture No."=w1214, "Test"="Striptest") -> ()  [unwired: 1 in, 2 out]
              n597 = One Button Dialog(message="Please switch bias off NOW and then open\nprobestation enclosure and raise needle.") -> ()  [unwired: 1 in, 1 out]
            }
            frame #3 {
              n598 = One Button Dialog(message="Please ensure detector bias is OFF!") -> ()  [unwired: 1 in, 1 out]
            }
          }
          n599 = case shown="True" w1093 {
            tunnel: [FALSE w1337] -> w1091
            frame False {
            }
            frame True {
              n600 = Two Button Dialog(message="Are you sure you don't want to save the data?", 1:"Quit" ("F button name (\"Cancel\")"), 2:"Save data" ("T button name (\"OK\")")) -> (T button?=w1337:bool)
            }
          }
          n601 = global read "ProbePlanParams.vi" "ProbePlan Parameters IN"() -> (w1090:T10)
          n602 = Unbundle By Name(w1090) -> ("Test ProbePoints.Regions Enabled"=w1088:bool[], "ProbePlan array"=w1087:T11)
          n603 = Array Size(array=w1088) -> (size(s)=w1089:i32)
          n604 = Or(x=w1092, y=w1091) -> (x .or. y?=w1081:bool)
          n605 = case shown="True" w1081 {
            tunnel: w1089 -> [w1237 w1265]
            tunnel: w1088 -> [w1236 w1264]
            tunnel: w1087 -> [_ w1263]
            tunnel: [w1232 w1261] -> w1084
            tunnel: [w1234 w1259] -> w1083
            tunnel: ["" w1256] -> w1082
            frame False {
              n606 = for {
                N: w1237 -> [_]
                tunnel: w1236 -> [w1241] mode=indexing
                tunnel: [w1240] -> w1235 mode=indexing
                tunnel: [w1239] -> w1233 mode=indexing
                i -> [w1238]
                n607 = case shown="True" w1241 {
                  tunnel: [100.0 w1246] -> w1240
                  tunnel: [TRUE w1245] -> w1239
                  tunnel: w1238 -> [_ w1244]
                  frame False {
                  }
                  frame True {
                    n608 = local read "probe points per region"() -> (w1252:i32[])
                    n609 = local read "max scale array"() -> (w1251:i32[])
                    n610 = local read "min scale array"() -> (w1250:i32[])
                    n611 = local read "Thresholds:"() -> (w1254:T2)
                    n612 = Index Array(array=w1252) -> (element=w1248:i32)  [unwired: 1 in]
                    n613 = call "DisplayStriptestData.vi"("min scale array"=w1250, "max scale array"=w1251, "# probed"=w1248, "Display Stats?"=TRUE, "Thresholds"=w1254, "Region"=w1244) -> ("Strip Quality Data"=w1249:T15)  [unwired: 4 out]
                    n614 = Unbundle By Name(w1249) -> ("pass Rate in %"=w1246:dbl)
                    n615 = Greater?(x=w1246, y=98.0) -> (0:w1245:bool)
                  }
                }
              }
              n616 = And Array Elements(Boolean array=w1233) -> (logical AND=w1232:bool)
              n617 = Array Max & Min(array=w1235) -> (min value=w1234:dbl)  [unwired: 3 out]
            }
            frame True {
              n618 = for {
                N: w1265 -> [_]
                tunnel: w1264 -> [w1275] mode=indexing
                tunnel: w1263 -> [w1274] mode=indexing
                tunnel: [w1272] -> w1262 mode=indexing
                tunnel: [w1271] -> w1260 mode=indexing
                tunnel: [w1270] -> w1258
                shift-right: [w1269] -> w1255
                shift-left: _ -> [w1266]
                i -> [w1273]
                n619 = case shown="True" w1275 {
                  tunnel: w1273 -> [_ w1288]
                  tunnel: w1274 -> [_ w1287]
                  tunnel: [TRUE w1284] -> w1272
                  tunnel: [100.0 w1282] -> w1271
                  tunnel: [w1276 w1281] -> w1270
                  tunnel: [w1276 w1280] -> w1267
                  frame False {
                    w1276 = ""
                  }
                  frame True {
                    n620 = Unbundle By Name(w1287) -> ("Region"=w1286:string)
                    n621 = flat-sequence {
                      tunnel: w1288 -> [w1312]
                      tunnel: w1286 -> [w1289]
                      tunnel: [w1312] -> w1285
                      tunnel: [w1313] -> w1283
                      tunnel: [w1291] -> w1281
                      tunnel: [w1290] -> w1280
                      tunnel: [w1289] -> w1279
                      tunnel: w1285 -> [w1324]
                      tunnel: [w1326] -> w1284
                      tunnel: w1283 -> [w1322]
                      tunnel: [w1323] -> w1282
                      tunnel: w1279 -> [w1321]
                      frame #0 {
                        w1306 = T17."Read Array" ("Action")
                        n622 = Concatenate Strings("Saving data for " ("string"), w1289) -> (w1319:string)
                        n623 = local write "Status:"(w1319) -> ()
                        n624 = call "MultiRegionData.vi"("Action"=w1306, "Array No."=4, "Region index"=w1312) -> ("Array OUT"=w1304:dbl[])  [unwired: 3 in, 1 out]
                        n625 = Multiply(x=w1304, y=0.001) -> (x*y=w1303:dbl[])
                        n626 = call "MultiRegionData.vi"("Action"=w1306, "Array No."=0, "Region index"=w1312) -> ("Array OUT"=w1299:dbl[])  [unwired: 3 in, 1 out]
                        n627 = call "MultiRegionData.vi"("Action"=w1306, "Array No."=1, "Region index"=w1312) -> ("Array OUT"=w1300:dbl[])  [unwired: 3 in, 1 out]
                        n628 = call "MultiRegionData.vi"("Action"=w1306, "Array No."=3, "Region index"=w1312) -> ("Array OUT"=w1302:dbl[])  [unwired: 3 in, 1 out]
                        n629 = local read "Temperature Progression"() -> (w1294:T3)
                        n630 = call "MultiRegionData.vi"("Array No."=2, "Region index"=w1312) -> ("Array OUT"=w1301:dbl[])  [unwired: 4 in, 1 out]
                        n631 = Build Array(w1299, w1300, w1301, w1302, w1303) -> (w1298:dbl[][])
                        n632 = Transpose 2D Array(2D array=w1298) -> (transposed array=w1297:dbl[][])
                        n633 = local read "probe points per region"() -> (w1320:i32[])
                        n634 = Unbundle By Name(w1294) -> ("Temperature Array [°C]"=w1293:dbl[], "Humidity Array [RH %]"=w1292:dbl[])
                        n635 = call <vilib>:"Std Deviation and Variance.vi"("X"=w1293) -> ("mean"=w1296:dbl)  [unwired: 1 in, 2 out]
                        n636 = call <vilib>:"Std Deviation and Variance.vi"("X"=w1292) -> ("mean"=w1295:dbl)  [unwired: 1 in, 2 out]
                        n637 = Index Array(array=w1320, index=w1312) -> (element=w1315:i32)
                        n638 = call "SaveDataFile.vi"("Data Array"=w1297, "Temperature"=w1296, "Humidity"=w1295, "no. of arrays"=5, "Actual array lengths"=w1315, "Array Titles"="ProbeplanIndex Current PinholeFlag Capacitance Resistance", "Strip Segment"=w1289, "Arrays format"="%016.6f") -> ("Filename OUT"=w1290:string, "Pathname OUT"=w1291:string, "Path + Filename OUT"=w1313:string)  [unwired: 4 in, 1 out]
                      }
                      frame #1 {
                        n639 = local read "probe points per region"() -> (w1333:i32[])
                        n640 = local read "max scale array"() -> (w1332:i32[])
                        n641 = local read "min scale array"() -> (w1331:i32[])
                        n642 = local read "Thresholds:"() -> (w1335:T2)
                        n643 = Index Array(array=w1333, index=w1324) -> (element=w1325:i32)
                        n644 = call "DisplayStriptestData.vi"("min scale array"=w1331, "max scale array"=w1332, "# probed"=w1325, "Display Stats?"=TRUE, "Thresholds"=w1335, "Region"=w1324) -> ("Strip Quality Data"=w1330:T15)  [unwired: 4 out]
                        n645 = Unbundle By Name(w1330) -> ("pass Rate in %"=w1323:dbl, "Bad channel list"=w1329:i32[], "No of bad strips"=w1328:i32, "Defect description list"=w1327:i32[])
                        n646 = call "CreateDefectFile.vi"("Segment:"=w1321, "Pass rate"=w1323, "Defect description list"=w1327, "Bad channel array"=w1329, "No of bad strips"=w1328, "Filename IN"=w1322) -> ("passed"=w1326:bool)  [unwired: 3 in, 2 out]
                      }
                    }
                  }
                }
                n647 = call <vilib>:"Space Constant.vi"() -> ("String"=w1268:string)
                n648 = Concatenate Strings(w1266, w1268, w1267) -> (w1269:string)
              }
              n649 = Array Max & Min(array=w1260) -> (min value=w1259:dbl)  [unwired: 3 out]
              n650 = And Array Elements(Boolean array=w1262) -> (logical AND=w1261:bool)
              "Module failed/passed" <- w1261
              n651 = call <vilib>:"Space Constant.vi"() -> ("String"=w1257:string)
              n652 = Concatenate Strings(w1258, w1257, w1255) -> (w1256:string)
            }
          }
          n653 = local read "Temperature Progression"() -> (w1080:T3)
          n654 = Unbundle By Name(w1080) -> ("Temperature Array [°C]"=w1078:dbl[], "Humidity Array [RH %]"=w1079:dbl[])
          n655 = call <vilib>:"Std Deviation and Variance.vi"("X"=w1078) -> ("standard deviation"=w1072:dbl)  [unwired: 1 in, 2 out]
          n656 = call <vilib>:"Std Deviation and Variance.vi"("X"=w1079) -> ("standard deviation"=w1071:dbl)  [unwired: 1 in, 2 out]
          n657 = Greater?(x=w1072, y=5) -> (0:w1069:bool)
          n658 = Greater?(x=w1071, y=10) -> (0:w1070:bool)
          n659 = Select(t="large temperature fluctuations", s=w1069, f=w1075) -> (s? t:f=w1066:string)
          n660 = Select(t="large humidity fluctuations", s=w1070, f=w1075) -> (s? t:f=w1067:string)
          n661 = Concatenate Strings(w1066, "\t", w1067) -> (w1065:string)
          n662 = call "WriteLogFile.vi"("Automatic warning"=w1065, "Data File"=w1082, "DUT passed?"=w1084, "Value TechSpec criteria"=w1083, "Files saved?"=w1081) -> ()  [unwired: 6 in, 1 out]
        }
      }
    }
  }
